vi "BS14P1.vi"() -> ()   [LabVIEW 2019]
doc: "Juego básico de Batalla naval implementado en TCP."
panel:
  out "String":string
  in  "Boolean 54":bool
  in  "Boolean 53":bool
  in  "Boolean 52":bool
  in  "Boolean 51":bool
  in  "?":bool
  out "error out":errorcluster
  in  "Boolean 50":bool
  in  "Boolean 49":bool
  in  "Boolean 48":bool
  in  "Boolean 47":bool
  in  "Boolean 46":bool
  in  "Boolean 45":bool
  in  "Boolean 44":bool
  in  "Boolean 43":bool
  in  "Boolean 42":bool
  in  "Boolean 41":bool
  in  "Boolean 40":bool
  in  "Boolean 39":bool
  in  "Boolean 38":bool
  in  "Boolean 37":bool
  in  "Boolean 36":bool
  in  "Boolean 35":bool
  in  "Boolean 34":bool
  in  "Boolean 33":bool
  in  "Boolean 32":bool
  in  "Boolean 31":bool
  in  "Boolean 30":bool
  in  "Boolean 29":bool
  in  "Boolean 28":bool
  in  "Boolean 27":bool
  in  "Boolean 26":bool
  in  "Boolean 25":bool
  in  "Boolean 24":bool
  in  "Boolean 23":bool
  in  "Boolean 22":bool
  in  "Boolean 21":bool
  in  "Boolean 20":bool
  in  "Boolean 19":bool
  in  "Boolean 18":bool
  in  "Boolean 17":bool
  in  "Boolean 16":bool
  in  "Boolean 15":bool
  in  "Boolean 14":bool
  in  "Boolean 13":bool
  in  "Boolean 12":bool
  in  "Boolean 11":bool
  in  "Boolean 10":bool
  in  "Boolean 9":bool
  in  "Boolean 8":bool
  in  "Boolean 7":bool
  in  "Boolean 6":bool
  in  "Boolean 5":bool
  in  "Boolean 4":bool
  in  "Boolean 3":bool
  in  "Boolean 2":bool
  in  "Boolean":bool
  # "Ship"
  # "Sea"
  # "Hit"
  # "Fail"
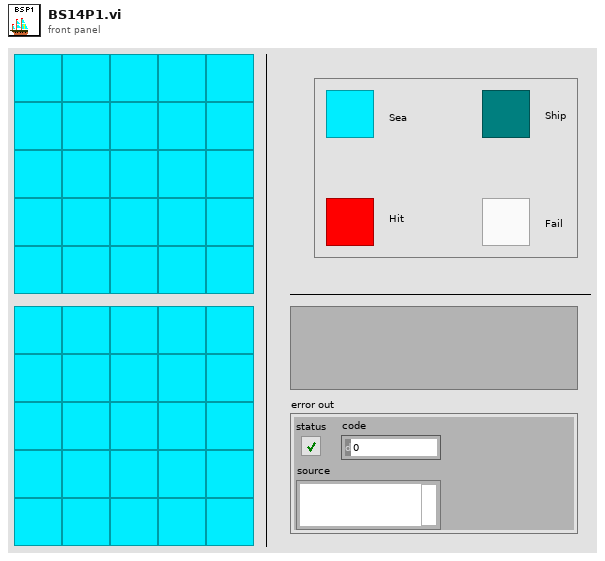
[diagram p1: front panel]
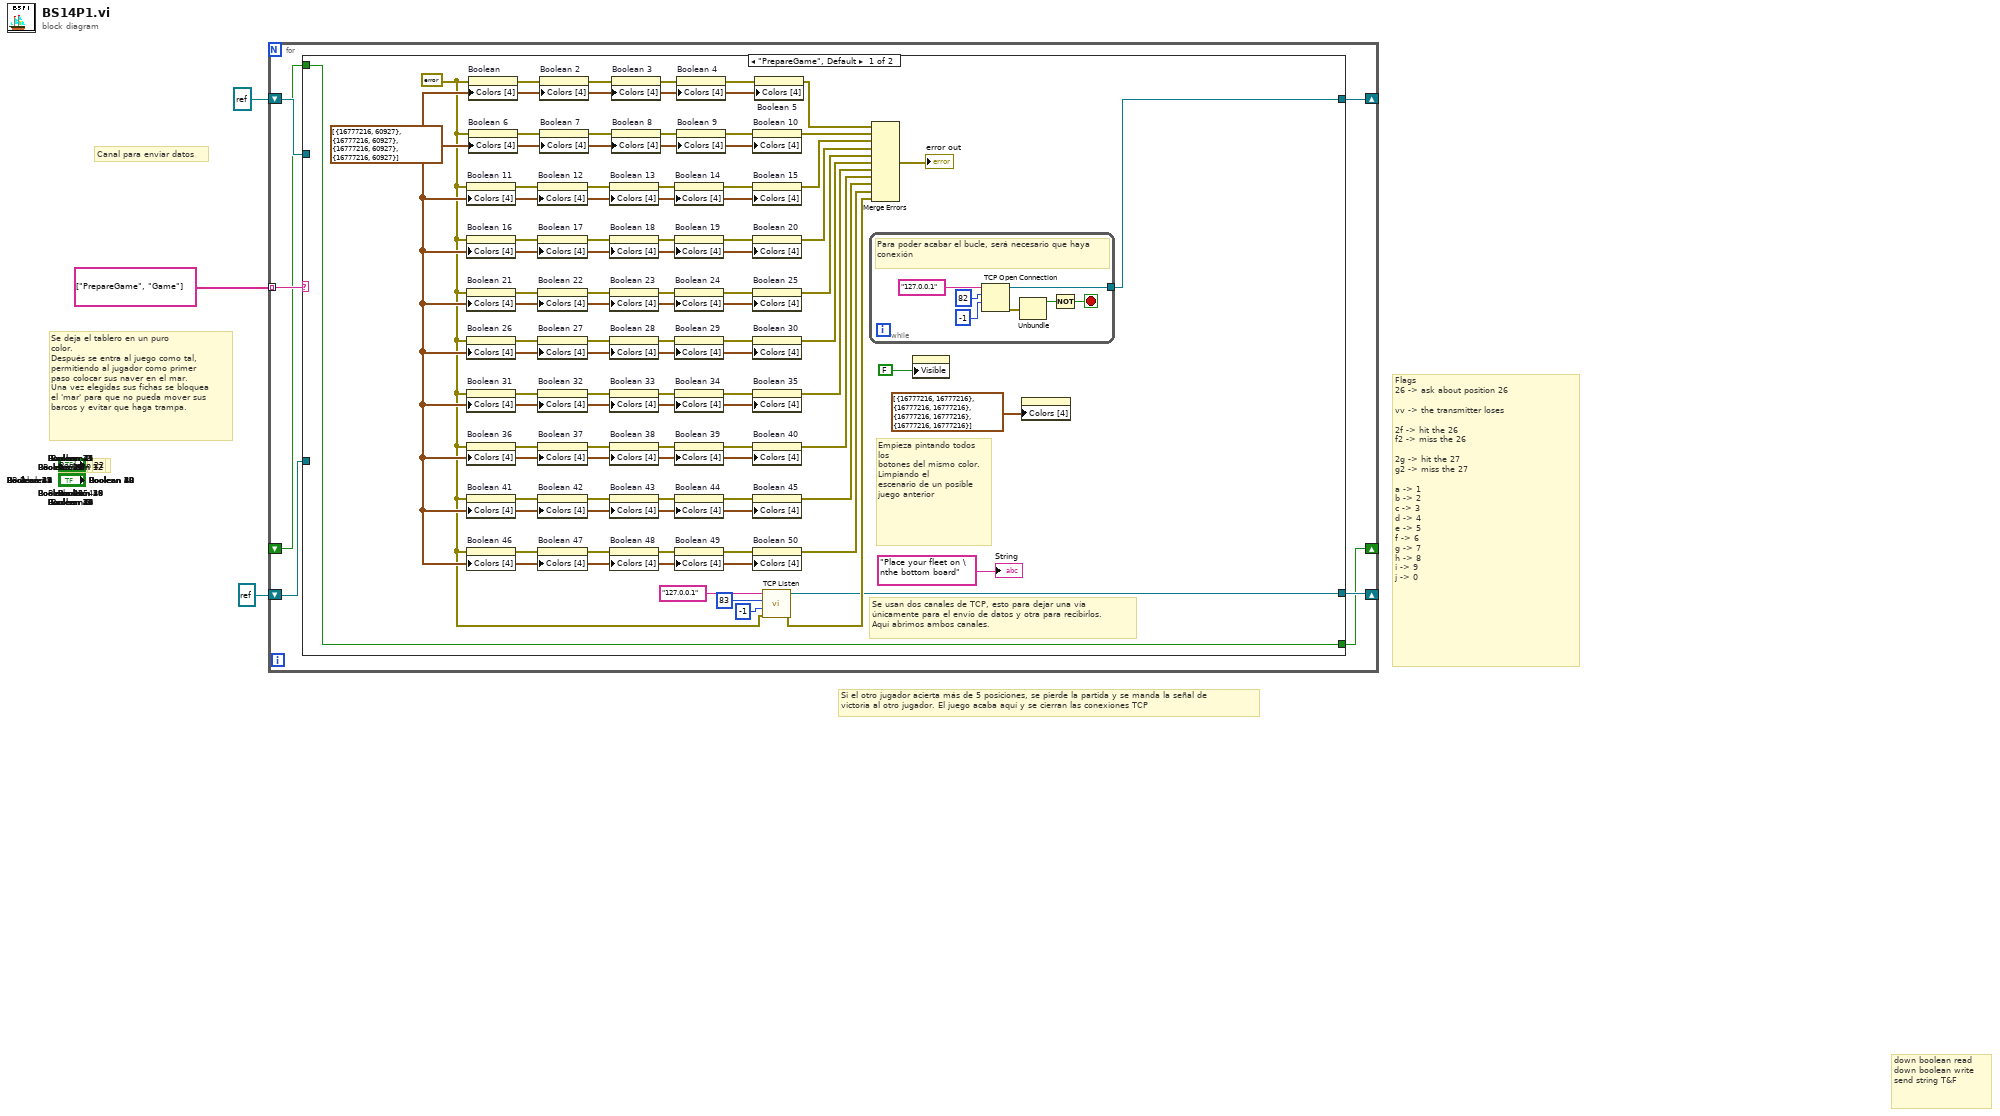
[diagram p0: block diagram]
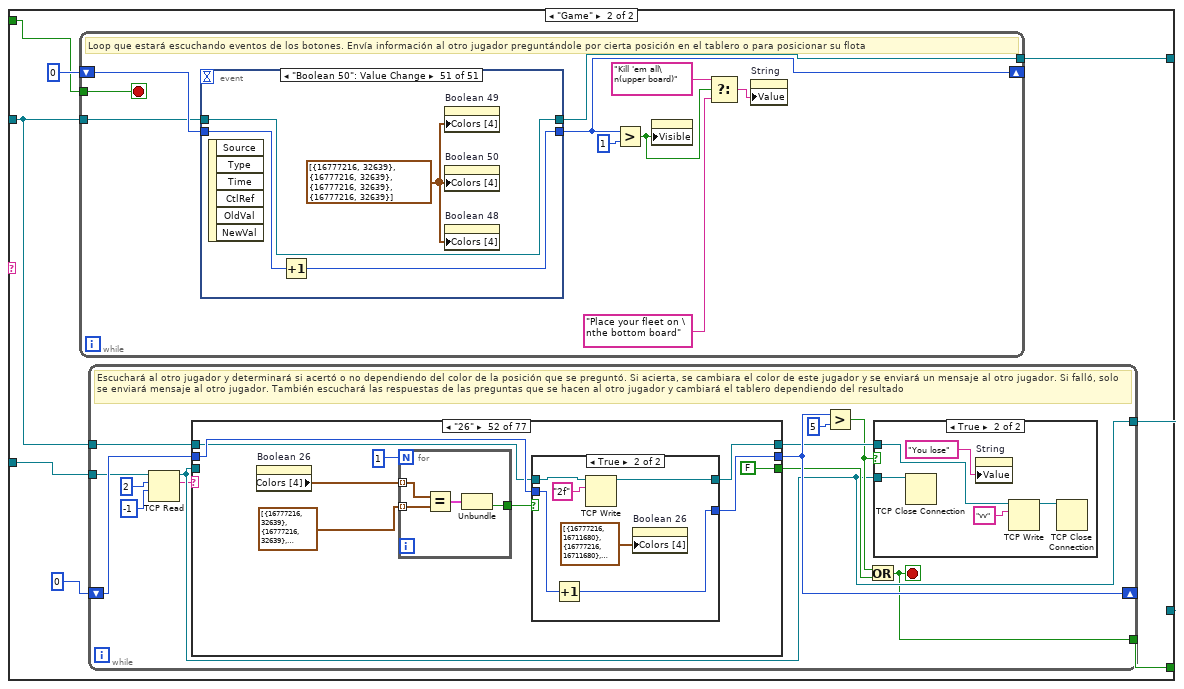
[diagram p2: hidden frame]
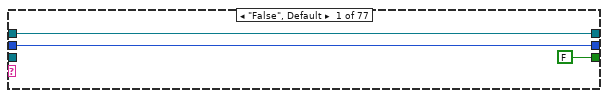
[diagram p3: hidden frame]
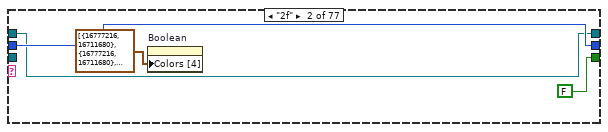
[diagram p4: hidden frame]
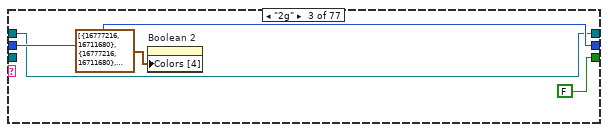
[diagram p5: hidden frame]
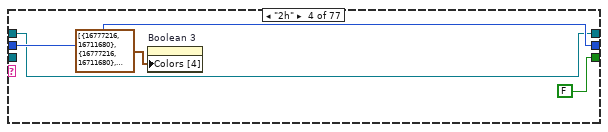
[diagram p6: hidden frame]
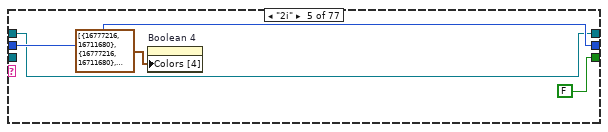
[diagram p7: hidden frame]
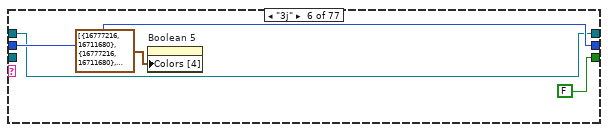
[diagram p8: hidden frame]
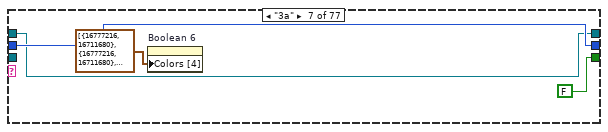
[diagram p9: hidden frame]
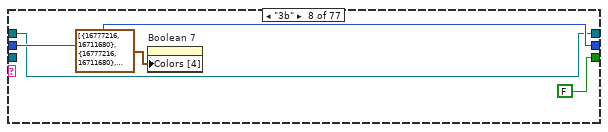
[diagram p10: hidden frame]
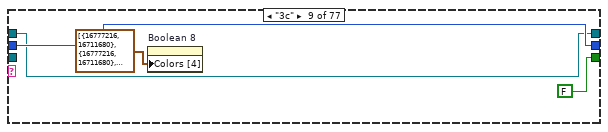
[diagram p11: hidden frame]
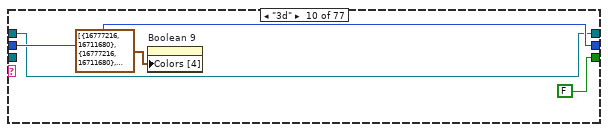
[diagram p12: hidden frame]
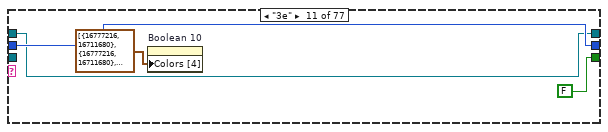
[diagram p13: hidden frame]
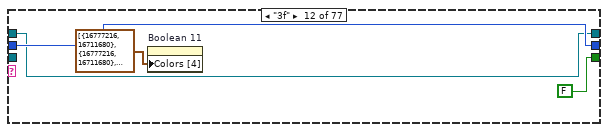
[diagram p14: hidden frame]
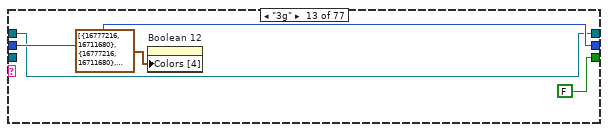
[diagram p15: hidden frame]
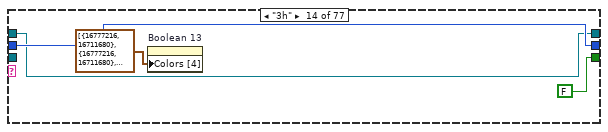
[diagram p16: hidden frame]
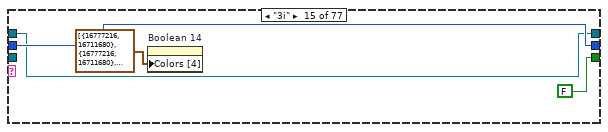
[diagram p17: hidden frame]
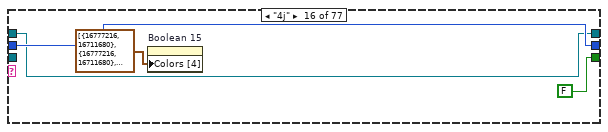
[diagram p18: hidden frame]
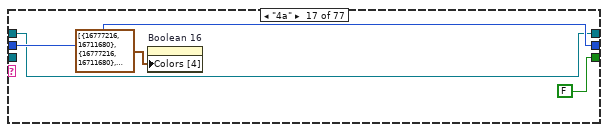
[diagram p19: hidden frame]
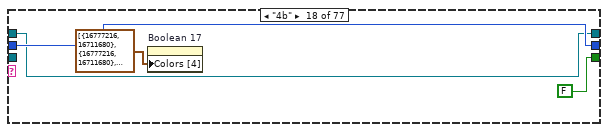
[diagram p20: hidden frame]
diagram:
  # "Si el otro jugador acierta más de 5 posiciones, se pierde la partida y se manda la señal de \nvictoria al otro jugador. El juego acaba aquí y se cierran las conexiones TCP"
  # "Canal para enviar datos"
  # "down boolean read\ndown boolean write \nsend string T&F"
  # "Flags\n26 -> ask about position 26\n\nvv -> the transmitter loses\n\n2f -> hit the 26\nf2 -> miss the 26\n\n2g -> hit the 27\ng2 -> miss the 27 \n\na -> 1\nb -> 2\nc -> 3\nd -> 4\ne -> 5 \nf -> 6 \ng -> 7\nh -> 8\ni -> 9\nj -> 0"
  # "Colors"
  # "block"
  # "Se deja el tablero en un puro \ncolor.\nDespués se entra al juego como tal,\npermitiendo al jugador como primer\npaso colocar sus naver en el mar. \nUna vez elegidas sus fichas se bloquea\nel 'mar' para que no pueda mover sus\nbarcos y evitar que haga trampa."
  # "inferiores"
  # "superiores"
  n1 = for {
    tunnel: string[] ["PrepareGame", "Game"] -> [w10] mode=indexing
    shift-right: [w9] -> _
    shift-left: refnum<k5> refnum ("connection ID") -> [w8]
    shift-right: [w7] -> _
    shift-left: refnum<k5> refnum ("connection ID out") -> [w6]
    shift-right: [w5] -> _
    shift-left: _ -> [w4]
    n2 = case shown="\"PrepareGame\", Default" w10 {
      tunnel: [w13 w84] -> w9
      tunnel: w8 -> [_ w86]
      tunnel: [w12 w85] -> w7
      tunnel: w6 -> [_ w83]
      tunnel: [w11 w82] -> w5
      tunnel: w4 -> [w11 w81]
      frame "PrepareGame", Default {
        w15 = errorcluster {"status"=FALSE, "code"=0, "source"=""} ("error in (no error)")
        w22 = cluster{u32, u32}[] [{16777216, 60927}, {16777216, 60927}, {16777216, 60927}, {16777216, 60927}] ("Colors [4] 2")
        # "Se usan dos canales de TCP, esto para dejar una vía \núnicamente para el envío de datos y otra para recibirlos.\nAquí abrimos ambos canales."
        # "Empieza pintando todos los \nbotones del mismo color. Limpiando el \nescenario de un posible juego anterior"
        n3 = property on="Boolean 11" class="Bool (strict)"(error in=w15, "Colors [4]"=w22) -> (error out=w58:errorcluster)  [unwired: 1 in, 1 out]
        n4 = property on="Boolean 16" class="Bool (strict)"(error in=w15, "Colors [4]"=w22) -> (error out=w56:errorcluster)  [unwired: 1 in, 1 out]
        n5 = property on="Boolean 21" class="Bool (strict)"(error in=w15, "Colors [4]"=w22) -> (error out=w55:errorcluster)  [unwired: 1 in, 1 out]
        n6 = property on="Boolean 26" class="Bool (strict)"(error in=w15, "Colors [4]"=w22) -> (error out=w47:errorcluster)  [unwired: 1 in, 1 out]
        n7 = property on="Boolean 31" class="Bool (strict)"(error in=w15, "Colors [4]"=w22) -> (error out=w43:errorcluster)  [unwired: 1 in, 1 out]
        n8 = property on="Boolean 36" class="Bool (strict)"(error in=w15, "Colors [4]"=w22) -> (error out=w39:errorcluster)  [unwired: 1 in, 1 out]
        n9 = property on="Boolean 41" class="Bool (strict)"(error in=w15, "Colors [4]"=w22) -> (error out=w35:errorcluster)  [unwired: 1 in, 1 out]
        n10 = property on="Boolean 46" class="Bool (strict)"(error in=w15, "Colors [4]"=w22) -> (error out=w31:errorcluster)  [unwired: 1 in, 1 out]
        n11 = property on="Boolean" class="Bool (strict)"(error in=w15, "Colors [4]"=w22) -> (error out=w66:errorcluster)  [unwired: 1 in, 1 out]
        n12 = property on="Boolean 6" class="Bool (strict)"(error in=w15, "Colors [4]"=w22) -> (error out=w62:errorcluster)  [unwired: 1 in, 1 out]
        n13 = property on="Boolean 12" class="Bool (strict)"(error in=w58, "Colors [4]"=w22) -> (error out=w57:errorcluster)  [unwired: 1 in, 1 out]
        n14 = property on="Boolean 17" class="Bool (strict)"(error in=w56, "Colors [4]"=w22) -> (error out=w71:errorcluster)  [unwired: 1 in, 1 out]
        n15 = property on="Boolean 22" class="Bool (strict)"(error in=w55, "Colors [4]"=w22) -> (error out=w68:errorcluster)  [unwired: 1 in, 1 out]
        n16 = property on="Boolean 27" class="Bool (strict)"(error in=w47, "Colors [4]"=w22) -> (error out=w46:errorcluster)  [unwired: 1 in, 1 out]
        n17 = property on="Boolean 32" class="Bool (strict)"(error in=w43, "Colors [4]"=w22) -> (error out=w42:errorcluster)  [unwired: 1 in, 1 out]
        n18 = property on="Boolean 37" class="Bool (strict)"(error in=w39, "Colors [4]"=w22) -> (error out=w38:errorcluster)  [unwired: 1 in, 1 out]
        n19 = property on="Boolean 42" class="Bool (strict)"(error in=w35, "Colors [4]"=w22) -> (error out=w34:errorcluster)  [unwired: 1 in, 1 out]
        n20 = property on="Boolean 47" class="Bool (strict)"(error in=w31, "Colors [4]"=w22) -> (error out=w30:errorcluster)  [unwired: 1 in, 1 out]
        n21 = property on="Boolean 2" class="Bool (strict)"(error in=w66, "Colors [4]"=w22) -> (error out=w65:errorcluster)  [unwired: 1 in, 1 out]
        n22 = property on="Boolean 7" class="Bool (strict)"(error in=w62, "Colors [4]"=w22) -> (error out=w61:errorcluster)  [unwired: 1 in, 1 out]
        n23 = property on="Boolean 13" class="Bool (strict)"(error in=w57, "Colors [4]"=w22) -> (error out=w73:errorcluster)  [unwired: 1 in, 1 out]
        n24 = property on="Boolean 18" class="Bool (strict)"(error in=w71, "Colors [4]"=w22) -> (error out=w70:errorcluster)  [unwired: 1 in, 1 out]
        n25 = property on="Boolean 23" class="Bool (strict)"(error in=w68, "Colors [4]"=w22) -> (error out=w67:errorcluster)  [unwired: 1 in, 1 out]
        n26 = property on="Boolean 28" class="Bool (strict)"(error in=w46, "Colors [4]"=w22) -> (error out=w45:errorcluster)  [unwired: 1 in, 1 out]
        n27 = property on="Boolean 33" class="Bool (strict)"(error in=w42, "Colors [4]"=w22) -> (error out=w41:errorcluster)  [unwired: 1 in, 1 out]
        n28 = property on="Boolean 38" class="Bool (strict)"(error in=w38, "Colors [4]"=w22) -> (error out=w37:errorcluster)  [unwired: 1 in, 1 out]
        n29 = property on="Boolean 43" class="Bool (strict)"(error in=w34, "Colors [4]"=w22) -> (error out=w33:errorcluster)  [unwired: 1 in, 1 out]
        n30 = property on="Boolean 48" class="Bool (strict)"(error in=w30, "Colors [4]"=w22) -> (error out=w29:errorcluster)  [unwired: 1 in, 1 out]
        n31 = property on="Boolean 3" class="Bool (strict)"(error in=w65, "Colors [4]"=w22) -> (error out=w64:errorcluster)  [unwired: 1 in, 1 out]
        n32 = property on="Boolean 8" class="Bool (strict)"(error in=w61, "Colors [4]"=w22) -> (error out=w60:errorcluster)  [unwired: 1 in, 1 out]
        n33 = property on="Boolean 14" class="Bool (strict)"(error in=w73, "Colors [4]"=w22) -> (error out=w72:errorcluster)  [unwired: 1 in, 1 out]
        n34 = property on="Boolean 19" class="Bool (strict)"(error in=w70, "Colors [4]"=w22) -> (error out=w69:errorcluster)  [unwired: 1 in, 1 out]
        n35 = property on="Boolean 24" class="Bool (strict)"(error in=w67, "Colors [4]"=w22) -> (error out=w54:errorcluster)  [unwired: 1 in, 1 out]
        n36 = property on="Boolean 29" class="Bool (strict)"(error in=w45, "Colors [4]"=w22) -> (error out=w44:errorcluster)  [unwired: 1 in, 1 out]
        n37 = property on="Boolean 34" class="Bool (strict)"(error in=w41, "Colors [4]"=w22) -> (error out=w40:errorcluster)  [unwired: 1 in, 1 out]
        n38 = property on="Boolean 39" class="Bool (strict)"(error in=w37, "Colors [4]"=w22) -> (error out=w36:errorcluster)  [unwired: 1 in, 1 out]
        n39 = property on="Boolean 44" class="Bool (strict)"(error in=w33, "Colors [4]"=w22) -> (error out=w32:errorcluster)  [unwired: 1 in, 1 out]
        n40 = property on="Boolean 49" class="Bool (strict)"(error in=w29, "Colors [4]"=w22) -> (error out=w28:errorcluster)  [unwired: 1 in, 1 out]
        n41 = property on="Boolean 4" class="Bool (strict)"(error in=w64, "Colors [4]"=w22) -> (error out=w63:errorcluster)  [unwired: 1 in, 1 out]
        n42 = property on="Boolean 9" class="Bool (strict)"(error in=w60, "Colors [4]"=w22) -> (error out=w59:errorcluster)  [unwired: 1 in, 1 out]
        n43 = property on="Boolean 10" class="Bool (strict)"(error in=w59, "Colors [4]"=w22) -> (error out=w51:errorcluster)  [unwired: 1 in, 1 out]
        n44 = property on="Boolean 15" class="Bool (strict)"(error in=w72, "Colors [4]"=w22) -> (error out=w50:errorcluster)  [unwired: 1 in, 1 out]
        n45 = property on="Boolean 20" class="Bool (strict)"(error in=w69, "Colors [4]"=w22) -> (error out=w49:errorcluster)  [unwired: 1 in, 1 out]
        n46 = property on="Boolean 25" class="Bool (strict)"(error in=w54, "Colors [4]"=w22) -> (error out=w48:errorcluster)  [unwired: 1 in, 1 out]
        n47 = property on="Boolean 30" class="Bool (strict)"(error in=w44, "Colors [4]"=w22) -> (error out=w27:errorcluster)  [unwired: 1 in, 1 out]
        n48 = property on="Boolean 35" class="Bool (strict)"(error in=w40, "Colors [4]"=w22) -> (error out=w26:errorcluster)  [unwired: 1 in, 1 out]
        n49 = property on="Boolean 40" class="Bool (strict)"(error in=w36, "Colors [4]"=w22) -> (error out=w25:errorcluster)  [unwired: 1 in, 1 out]
        n50 = property on="Boolean 45" class="Bool (strict)"(error in=w32, "Colors [4]"=w22) -> (error out=w24:errorcluster)  [unwired: 1 in, 1 out]
        n51 = property on="Boolean 50" class="Bool (strict)"(error in=w28, "Colors [4]"=w22) -> (error out=w23:errorcluster)  [unwired: 1 in, 1 out]
        n52 = property on="Boolean 5" class="Bool (strict)"(error in=w63, "Colors [4]"=w22) -> (error out=w53:errorcluster)  [unwired: 1 in, 1 out]
        n53 = call <vilib>:"TCP Listen.vi"("error in (no error)"=w15, "timeout ms (wait forever: -1)"=-1, "port"=u16 83, "service name"="127.0.0.1") -> ("error out"=w14:errorcluster, "connection ID"=w13:refnum<k5>)  [unwired: 3 in, 3 out]
        n54 = while {
          tunnel: [w74] -> w12
          stop <- w75 stop-if-true
          # "Para poder acabar el bucle, será necesario que haya conexión"
          n55 = TCP Open Connection(address="127.0.0.1", remote port or service name=u16 82, timeout ms (60000)=-1) -> (connection ID=w74:refnum<k5>, error out=w76:errorcluster)  [unwired: 2 in]
          n56 = Unbundle(w76) -> ("status"=w77:bool)  [unwired: 2 out]
          n57 = Not(x=w77) -> (.not. x?=w75:bool)
        }
        n58 = Merge Errors(w53, w51, w50, w49, w48, w27, w26, w25, w24, w23, w14) -> (→"error out":errorcluster)
        n59 = property class="Bool (strict)"("Visible"=FALSE) -> ()  [unwired: 2 in, 2 out]
        n60 = property class="Bool (strict)"("Colors [4]"=cluster{u32, u32}[] [{16777216, 16777216}, {16777216, 16777216}, {16777216, 16777216}, {16777216, 16777216}] ("Colors [4] 2")) -> ()  [unwired: 2 in, 2 out]
        "String" <- "Place your fleet on \nthe bottom board"
      }
      frame "Game" {
        n61 = while {
          shift-right: [w898] -> _
          shift-left: 0 -> [w899]
          tunnel: w83 -> [w892]
          tunnel: [w891] -> w85
          tunnel: w81 -> [w890]
          stop <- w890 stop-if-true
          # "Loop que estará escuchando eventos de los botones. Envía información al otro jugador preguntándole por cierta posición en el tablero o para posicionar su flota"
          n62 = event shown="[50] \"Boolean 50\": Value Change" {
            selector: _ -> [_ _ _ _ _ _ _ _ _ _ _ _ _ _ _ _ _ _ _ _ _ _ _ _ _ _ _ _ _ _ _ _ _ _ _ _ _ _ _ _ _ _ _ _ _ _ _ _ _ _ _]
            dyn-events: _ -> [_ _ _ _ _ _ _ _ _ _ _ _ _ _ _ _ _ _ _ _ _ _ _ _ _ _ _ _ _ _ _ _ _ _ _ _ _ _ _ _ _ _ _ _ _ _ _ _ _ _ _]
            timeout: _ -> [_ _ _ _ _ _ _ _ _ _ _ _ _ _ _ _ _ _ _ _ _ _ _ _ _ _ _ _ _ _ _ _ _ _ _ _ _ _ _ _ _ _ _ _ _ _ _ _ _ _ _]
            tunnel: w899 -> [w901 w905 w909 w913 w917 w921 w925 w929 w933 w937 w941 w945 w949 w953 w957 w961 w965 w969 w973 w977 w981 w985 w989 w993 w997 w1001 w1004 w1008 w1012 w1016 w1020 w1024 w1028 w1032 w1036 w1040 w1044 w1048 w1052 w1056 w1060 w1064 w1068 w1072 w1076 w1080 w1084 w1088 w1092 w1096 w1100]
            tunnel: [w901 w905 w909 w913 w917 w921 w925 w929 w933 w937 w941 w945 w949 w953 w957 w961 w965 w969 w973 w977 w981 w985 w989 w993 w997 w1001 w1003 w1007 w1011 w1015 w1019 w1023 w1027 w1031 w1035 w1039 w1043 w1047 w1051 w1055 w1059 w1063 w1067 w1071 w1075 w1079 w1083 w1087 w1091 w1095 w1099] -> w898
            tunnel: w892 -> [w900 w903 w907 w911 w915 w919 w923 w927 w931 w935 w939 w943 w947 w951 w955 w959 w963 w967 w971 w975 w979 w983 w987 w991 w995 w999 w1002 w1006 w1010 w1014 w1018 w1022 w1026 w1030 w1034 w1038 w1042 w1046 w1050 w1054 w1058 w1062 w1066 w1070 w1074 w1078 w1082 w1086 w1090 w1094 w1098]
            tunnel: [w900 w902 w906 w910 w914 w918 w922 w926 w930 w934 w938 w942 w946 w950 w954 w958 w962 w966 w970 w974 w978 w982 w986 w990 w994 w998 w1002 w1006 w1010 w1014 w1018 w1022 w1026 w1030 w1034 w1038 w1042 w1046 w1050 w1054 w1058 w1062 w1066 w1070 w1074 w1078 w1082 w1086 w1090 w1094 w1098] -> w891
            event Timeout {
              n63 = event-data() -> ()  [unwired: 1 in, 3 out]
            }
            event "Boolean": Value Change {
              n64 = event-data() -> ()  [unwired: 1 in, 6 out]
              n65 = TCP Write(connection ID=w903, data in="26") -> (connection ID out=w902:refnum<k5>)  [unwired: 2 in, 2 out]
            }
            event "Boolean 2": Value Change {
              n66 = event-data() -> ()  [unwired: 1 in, 6 out]
              n67 = TCP Write(connection ID=w907, data in="27") -> (connection ID out=w906:refnum<k5>)  [unwired: 2 in, 2 out]
            }
            event "Boolean 3": Value Change {
              n68 = event-data() -> ()  [unwired: 1 in, 6 out]
              n69 = TCP Write(connection ID=w911, data in="28") -> (connection ID out=w910:refnum<k5>)  [unwired: 2 in, 2 out]
            }
            event "Boolean 4": Value Change {
              n70 = event-data() -> ()  [unwired: 1 in, 6 out]
              n71 = TCP Write(connection ID=w915, data in="29") -> (connection ID out=w914:refnum<k5>)  [unwired: 2 in, 2 out]
            }
            event "Boolean 5": Value Change {
              n72 = event-data() -> ()  [unwired: 1 in, 6 out]
              n73 = TCP Write(connection ID=w919, data in="30") -> (connection ID out=w918:refnum<k5>)  [unwired: 2 in, 2 out]
            }
            event "Boolean 6": Value Change {
              n74 = event-data() -> ()  [unwired: 1 in, 6 out]
              n75 = TCP Write(connection ID=w923, data in="31") -> (connection ID out=w922:refnum<k5>)  [unwired: 2 in, 2 out]
            }
            event "Boolean 7": Value Change {
              n76 = event-data() -> ()  [unwired: 1 in, 6 out]
              n77 = TCP Write(connection ID=w927, data in="32") -> (connection ID out=w926:refnum<k5>)  [unwired: 2 in, 2 out]
            }
            event "Boolean 8": Value Change {
              n78 = event-data() -> ()  [unwired: 1 in, 6 out]
              n79 = TCP Write(connection ID=w931, data in="33") -> (connection ID out=w930:refnum<k5>)  [unwired: 2 in, 2 out]
            }
            event "Boolean 9": Value Change {
              n80 = event-data() -> ()  [unwired: 1 in, 6 out]
              n81 = TCP Write(connection ID=w935, data in="34") -> (connection ID out=w934:refnum<k5>)  [unwired: 2 in, 2 out]
            }
            event "Boolean 10": Value Change {
              n82 = event-data() -> ()  [unwired: 1 in, 6 out]
              n83 = TCP Write(connection ID=w939, data in="35") -> (connection ID out=w938:refnum<k5>)  [unwired: 2 in, 2 out]
            }
            event "Boolean 11": Value Change {
              n84 = event-data() -> ()  [unwired: 1 in, 6 out]
              n85 = TCP Write(connection ID=w943, data in="36") -> (connection ID out=w942:refnum<k5>)  [unwired: 2 in, 2 out]
            }
            event "Boolean 12": Value Change {
              n86 = event-data() -> ()  [unwired: 1 in, 6 out]
              n87 = TCP Write(connection ID=w947, data in="37") -> (connection ID out=w946:refnum<k5>)  [unwired: 2 in, 2 out]
            }
            event "Boolean 13": Value Change {
              n88 = event-data() -> ()  [unwired: 1 in, 6 out]
              n89 = TCP Write(connection ID=w951, data in="38") -> (connection ID out=w950:refnum<k5>)  [unwired: 2 in, 2 out]
            }
            event "Boolean 14": Value Change {
              n90 = event-data() -> ()  [unwired: 1 in, 6 out]
              n91 = TCP Write(connection ID=w955, data in="39") -> (connection ID out=w954:refnum<k5>)  [unwired: 2 in, 2 out]
            }
            event "Boolean 15": Value Change {
              n92 = event-data() -> ()  [unwired: 1 in, 6 out]
              n93 = TCP Write(connection ID=w959, data in="40") -> (connection ID out=w958:refnum<k5>)  [unwired: 2 in, 2 out]
            }
            event "Boolean 16": Value Change {
              n94 = event-data() -> ()  [unwired: 1 in, 6 out]
              n95 = TCP Write(connection ID=w963, data in="41") -> (connection ID out=w962:refnum<k5>)  [unwired: 2 in, 2 out]
            }
            event "Boolean 17": Value Change {
              n96 = event-data() -> ()  [unwired: 1 in, 6 out]
              n97 = TCP Write(connection ID=w967, data in="42") -> (connection ID out=w966:refnum<k5>)  [unwired: 2 in, 2 out]
            }
            event "Boolean 18": Value Change {
              n98 = event-data() -> ()  [unwired: 1 in, 6 out]
              n99 = TCP Write(connection ID=w971, data in="43") -> (connection ID out=w970:refnum<k5>)  [unwired: 2 in, 2 out]
            }
            event "Boolean 19": Value Change {
              n100 = event-data() -> ()  [unwired: 1 in, 6 out]
              n101 = TCP Write(connection ID=w975, data in="44") -> (connection ID out=w974:refnum<k5>)  [unwired: 2 in, 2 out]
            }
            event "Boolean 20": Value Change {
              n102 = event-data() -> ()  [unwired: 1 in, 6 out]
              n103 = TCP Write(connection ID=w979, data in="45") -> (connection ID out=w978:refnum<k5>)  [unwired: 2 in, 2 out]
            }
            event "Boolean 21": Value Change {
              n104 = event-data() -> ()  [unwired: 1 in, 6 out]
              n105 = TCP Write(connection ID=w983, data in="46") -> (connection ID out=w982:refnum<k5>)  [unwired: 2 in, 2 out]
            }
            event "Boolean 22": Value Change {
              n106 = event-data() -> ()  [unwired: 1 in, 6 out]
              n107 = TCP Write(connection ID=w987, data in="47") -> (connection ID out=w986:refnum<k5>)  [unwired: 2 in, 2 out]
            }
            event "Boolean 23": Value Change {
              n108 = event-data() -> ()  [unwired: 1 in, 6 out]
              n109 = TCP Write(connection ID=w991, data in="48") -> (connection ID out=w990:refnum<k5>)  [unwired: 2 in, 2 out]
            }
            event "Boolean 24": Value Change {
              n110 = event-data() -> ()  [unwired: 1 in, 6 out]
              n111 = TCP Write(connection ID=w995, data in="49") -> (connection ID out=w994:refnum<k5>)  [unwired: 2 in, 2 out]
            }
            event "Boolean 25": Value Change {
              n112 = event-data() -> ()  [unwired: 1 in, 6 out]
              n113 = TCP Write(connection ID=w999, data in="50") -> (connection ID out=w998:refnum<k5>)  [unwired: 2 in, 2 out]
            }
            event "Boolean 26": Value Change {
              w1005 = cluster{u32, u32}[] [{16777216, 32639}, {16777216, 32639}, {16777216, 32639}, {16777216, 32639}] ("Colors [4] 2")
              n114 = event-data() -> ()  [unwired: 1 in, 6 out]
              n115 = Increment(x=w1004) -> (x+1=w1003:i32)
              n116 = property on="Boolean 27" class="Bool (strict)"("Colors [4]"=w1005) -> ()  [unwired: 2 in, 2 out]
              n117 = property on="Boolean 28" class="Bool (strict)"("Colors [4]"=w1005) -> ()  [unwired: 2 in, 2 out]
              n118 = property on="Boolean 26" class="Bool (strict)"("Colors [4]"=w1005) -> ()  [unwired: 2 in, 2 out]
            }
            event "Boolean 27": Value Change {
              w1009 = cluster{u32, u32}[] [{16777216, 32639}, {16777216, 32639}, {16777216, 32639}, {16777216, 32639}] ("Colors [4] 2")
              n119 = event-data() -> ()  [unwired: 1 in, 6 out]
              n120 = Increment(x=w1008) -> (x+1=w1007:i32)
              n121 = property on="Boolean 27" class="Bool (strict)"("Colors [4]"=w1009) -> ()  [unwired: 2 in, 2 out]
              n122 = property on="Boolean 28" class="Bool (strict)"("Colors [4]"=w1009) -> ()  [unwired: 2 in, 2 out]
              n123 = property on="Boolean 26" class="Bool (strict)"("Colors [4]"=w1009) -> ()  [unwired: 2 in, 2 out]
            }
            event "Boolean 28": Value Change {
              w1013 = cluster{u32, u32}[] [{16777216, 32639}, {16777216, 32639}, {16777216, 32639}, {16777216, 32639}] ("Colors [4] 2")
              n124 = event-data() -> ()  [unwired: 1 in, 6 out]
              n125 = Increment(x=w1012) -> (x+1=w1011:i32)
              n126 = property on="Boolean 29" class="Bool (strict)"("Colors [4]"=w1013) -> ()  [unwired: 2 in, 2 out]
              n127 = property on="Boolean 27" class="Bool (strict)"("Colors [4]"=w1013) -> ()  [unwired: 2 in, 2 out]
              n128 = property on="Boolean 28" class="Bool (strict)"("Colors [4]"=w1013) -> ()  [unwired: 2 in, 2 out]
            }
            event "Boolean 29": Value Change {
              w1017 = cluster{u32, u32}[] [{16777216, 32639}, {16777216, 32639}, {16777216, 32639}, {16777216, 32639}] ("Colors [4] 2")
              n129 = event-data() -> ()  [unwired: 1 in, 6 out]
              n130 = Increment(x=w1016) -> (x+1=w1015:i32)
              n131 = property on="Boolean 29" class="Bool (strict)"("Colors [4]"=w1017) -> ()  [unwired: 2 in, 2 out]
              n132 = property on="Boolean 30" class="Bool (strict)"("Colors [4]"=w1017) -> ()  [unwired: 2 in, 2 out]
              n133 = property on="Boolean 28" class="Bool (strict)"("Colors [4]"=w1017) -> ()  [unwired: 2 in, 2 out]
            }
            event "Boolean 30": Value Change {
              w1021 = cluster{u32, u32}[] [{16777216, 32639}, {16777216, 32639}, {16777216, 32639}, {16777216, 32639}] ("Colors [4] 2")
              n134 = event-data() -> ()  [unwired: 1 in, 6 out]
              n135 = Increment(x=w1020) -> (x+1=w1019:i32)
              n136 = property on="Boolean 29" class="Bool (strict)"("Colors [4]"=w1021) -> ()  [unwired: 2 in, 2 out]
              n137 = property on="Boolean 30" class="Bool (strict)"("Colors [4]"=w1021) -> ()  [unwired: 2 in, 2 out]
              n138 = property on="Boolean 28" class="Bool (strict)"("Colors [4]"=w1021) -> ()  [unwired: 2 in, 2 out]
            }
            event "Boolean 31": Value Change {
              w1025 = cluster{u32, u32}[] [{16777216, 32639}, {16777216, 32639}, {16777216, 32639}, {16777216, 32639}] ("Colors [4] 2")
              n139 = event-data() -> ()  [unwired: 1 in, 6 out]
              n140 = Increment(x=w1024) -> (x+1=w1023:i32)
              n141 = property on="Boolean 31" class="Bool (strict)"("Colors [4]"=w1025) -> ()  [unwired: 2 in, 2 out]
              n142 = property on="Boolean 32" class="Bool (strict)"("Colors [4]"=w1025) -> ()  [unwired: 2 in, 2 out]
              n143 = property on="Boolean 33" class="Bool (strict)"("Colors [4]"=w1025) -> ()  [unwired: 2 in, 2 out]
            }
            event "Boolean 32": Value Change {
              w1029 = cluster{u32, u32}[] [{16777216, 32639}, {16777216, 32639}, {16777216, 32639}, {16777216, 32639}] ("Colors [4] 2")
              n144 = event-data() -> ()  [unwired: 1 in, 6 out]
              n145 = Increment(x=w1028) -> (x+1=w1027:i32)
              n146 = property on="Boolean 31" class="Bool (strict)"("Colors [4]"=w1029) -> ()  [unwired: 2 in, 2 out]
              n147 = property on="Boolean 32" class="Bool (strict)"("Colors [4]"=w1029) -> ()  [unwired: 2 in, 2 out]
              n148 = property on="Boolean 33" class="Bool (strict)"("Colors [4]"=w1029) -> ()  [unwired: 2 in, 2 out]
            }
            event "Boolean 33": Value Change {
              w1033 = cluster{u32, u32}[] [{16777216, 32639}, {16777216, 32639}, {16777216, 32639}, {16777216, 32639}] ("Colors [4] 2")
              n149 = event-data() -> ()  [unwired: 1 in, 6 out]
              n150 = Increment(x=w1032) -> (x+1=w1031:i32)
              n151 = property on="Boolean 34" class="Bool (strict)"("Colors [4]"=w1033) -> ()  [unwired: 2 in, 2 out]
              n152 = property on="Boolean 32" class="Bool (strict)"("Colors [4]"=w1033) -> ()  [unwired: 2 in, 2 out]
              n153 = property on="Boolean 33" class="Bool (strict)"("Colors [4]"=w1033) -> ()  [unwired: 2 in, 2 out]
            }
            event "Boolean 34": Value Change {
              w1037 = cluster{u32, u32}[] [{16777216, 32639}, {16777216, 32639}, {16777216, 32639}, {16777216, 32639}] ("Colors [4] 2")
              n154 = event-data() -> ()  [unwired: 1 in, 6 out]
              n155 = Increment(x=w1036) -> (x+1=w1035:i32)
              n156 = property on="Boolean 34" class="Bool (strict)"("Colors [4]"=w1037) -> ()  [unwired: 2 in, 2 out]
              n157 = property on="Boolean 35" class="Bool (strict)"("Colors [4]"=w1037) -> ()  [unwired: 2 in, 2 out]
              n158 = property on="Boolean 33" class="Bool (strict)"("Colors [4]"=w1037) -> ()  [unwired: 2 in, 2 out]
            }
            event "Boolean 35": Value Change {
              w1041 = cluster{u32, u32}[] [{16777216, 32639}, {16777216, 32639}, {16777216, 32639}, {16777216, 32639}] ("Colors [4] 2")
              n159 = event-data() -> ()  [unwired: 1 in, 6 out]
              n160 = Increment(x=w1040) -> (x+1=w1039:i32)
              n161 = property on="Boolean 34" class="Bool (strict)"("Colors [4]"=w1041) -> ()  [unwired: 2 in, 2 out]
              n162 = property on="Boolean 35" class="Bool (strict)"("Colors [4]"=w1041) -> ()  [unwired: 2 in, 2 out]
              n163 = property on="Boolean 33" class="Bool (strict)"("Colors [4]"=w1041) -> ()  [unwired: 2 in, 2 out]
            }
            event "Boolean 36": Value Change {
              w1045 = cluster{u32, u32}[] [{16777216, 32639}, {16777216, 32639}, {16777216, 32639}, {16777216, 32639}] ("Colors [4] 2")
              n164 = event-data() -> ()  [unwired: 1 in, 6 out]
              n165 = Increment(x=w1044) -> (x+1=w1043:i32)
              n166 = property on="Boolean 37" class="Bool (strict)"("Colors [4]"=w1045) -> ()  [unwired: 2 in, 2 out]
              n167 = property on="Boolean 38" class="Bool (strict)"("Colors [4]"=w1045) -> ()  [unwired: 2 in, 2 out]
              n168 = property on="Boolean 36" class="Bool (strict)"("Colors [4]"=w1045) -> ()  [unwired: 2 in, 2 out]
            }
            event "Boolean 37": Value Change {
              w1049 = cluster{u32, u32}[] [{16777216, 32639}, {16777216, 32639}, {16777216, 32639}, {16777216, 32639}] ("Colors [4] 2")
              n169 = event-data() -> ()  [unwired: 1 in, 6 out]
              n170 = Increment(x=w1048) -> (x+1=w1047:i32)
              n171 = property on="Boolean 37" class="Bool (strict)"("Colors [4]"=w1049) -> ()  [unwired: 2 in, 2 out]
              n172 = property on="Boolean 38" class="Bool (strict)"("Colors [4]"=w1049) -> ()  [unwired: 2 in, 2 out]
              n173 = property on="Boolean 36" class="Bool (strict)"("Colors [4]"=w1049) -> ()  [unwired: 2 in, 2 out]
            }
            event "Boolean 38": Value Change {
              w1053 = cluster{u32, u32}[] [{16777216, 32639}, {16777216, 32639}, {16777216, 32639}, {16777216, 32639}] ("Colors [4] 2")
              n174 = event-data() -> ()  [unwired: 1 in, 6 out]
              n175 = Increment(x=w1052) -> (x+1=w1051:i32)
              n176 = property on="Boolean 39" class="Bool (strict)"("Colors [4]"=w1053) -> ()  [unwired: 2 in, 2 out]
              n177 = property on="Boolean 38" class="Bool (strict)"("Colors [4]"=w1053) -> ()  [unwired: 2 in, 2 out]
              n178 = property on="Boolean 37" class="Bool (strict)"("Colors [4]"=w1053) -> ()  [unwired: 2 in, 2 out]
            }
            event "Boolean 39": Value Change {
              w1057 = cluster{u32, u32}[] [{16777216, 32639}, {16777216, 32639}, {16777216, 32639}, {16777216, 32639}] ("Colors [4] 2")
              n179 = event-data() -> ()  [unwired: 1 in, 6 out]
              n180 = Increment(x=w1056) -> (x+1=w1055:i32)
              n181 = property on="Boolean 39" class="Bool (strict)"("Colors [4]"=w1057) -> ()  [unwired: 2 in, 2 out]
              n182 = property on="Boolean 40" class="Bool (strict)"("Colors [4]"=w1057) -> ()  [unwired: 2 in, 2 out]
              n183 = property on="Boolean 38" class="Bool (strict)"("Colors [4]"=w1057) -> ()  [unwired: 2 in, 2 out]
            }
            event "Boolean 40": Value Change {
              w1061 = cluster{u32, u32}[] [{16777216, 32639}, {16777216, 32639}, {16777216, 32639}, {16777216, 32639}] ("Colors [4] 2")
              n184 = event-data() -> ()  [unwired: 1 in, 6 out]
              n185 = Increment(x=w1060) -> (x+1=w1059:i32)
              n186 = property on="Boolean 39" class="Bool (strict)"("Colors [4]"=w1061) -> ()  [unwired: 2 in, 2 out]
              n187 = property on="Boolean 40" class="Bool (strict)"("Colors [4]"=w1061) -> ()  [unwired: 2 in, 2 out]
              n188 = property on="Boolean 38" class="Bool (strict)"("Colors [4]"=w1061) -> ()  [unwired: 2 in, 2 out]
            }
            event "Boolean 41": Value Change {
              w1065 = cluster{u32, u32}[] [{16777216, 32639}, {16777216, 32639}, {16777216, 32639}, {16777216, 32639}] ("Colors [4] 2")
              n189 = event-data() -> ()  [unwired: 1 in, 6 out]
              n190 = Increment(x=w1064) -> (x+1=w1063:i32)
              n191 = property on="Boolean 42" class="Bool (strict)"("Colors [4]"=w1065) -> ()  [unwired: 2 in, 2 out]
              n192 = property on="Boolean 43" class="Bool (strict)"("Colors [4]"=w1065) -> ()  [unwired: 2 in, 2 out]
              n193 = property on="Boolean 41" class="Bool (strict)"("Colors [4]"=w1065) -> ()  [unwired: 2 in, 2 out]
            }
            event "Boolean 42": Value Change {
              w1069 = cluster{u32, u32}[] [{16777216, 32639}, {16777216, 32639}, {16777216, 32639}, {16777216, 32639}] ("Colors [4] 2")
              n194 = event-data() -> ()  [unwired: 1 in, 6 out]
              n195 = Increment(x=w1068) -> (x+1=w1067:i32)
              n196 = property on="Boolean 42" class="Bool (strict)"("Colors [4]"=w1069) -> ()  [unwired: 2 in, 2 out]
              n197 = property on="Boolean 43" class="Bool (strict)"("Colors [4]"=w1069) -> ()  [unwired: 2 in, 2 out]
              n198 = property on="Boolean 41" class="Bool (strict)"("Colors [4]"=w1069) -> ()  [unwired: 2 in, 2 out]
            }
            event "Boolean 43": Value Change {
              w1073 = cluster{u32, u32}[] [{16777216, 32639}, {16777216, 32639}, {16777216, 32639}, {16777216, 32639}] ("Colors [4] 2")
              n199 = event-data() -> ()  [unwired: 1 in, 6 out]
              n200 = Increment(x=w1072) -> (x+1=w1071:i32)
              n201 = property on="Boolean 44" class="Bool (strict)"("Colors [4]"=w1073) -> ()  [unwired: 2 in, 2 out]
              n202 = property on="Boolean 43" class="Bool (strict)"("Colors [4]"=w1073) -> ()  [unwired: 2 in, 2 out]
              n203 = property on="Boolean 42" class="Bool (strict)"("Colors [4]"=w1073) -> ()  [unwired: 2 in, 2 out]
            }
            event "Boolean 44": Value Change {
              w1077 = cluster{u32, u32}[] [{16777216, 32639}, {16777216, 32639}, {16777216, 32639}, {16777216, 32639}] ("Colors [4] 2")
              n204 = event-data() -> ()  [unwired: 1 in, 6 out]
              n205 = Increment(x=w1076) -> (x+1=w1075:i32)
              n206 = property on="Boolean 44" class="Bool (strict)"("Colors [4]"=w1077) -> ()  [unwired: 2 in, 2 out]
              n207 = property on="Boolean 45" class="Bool (strict)"("Colors [4]"=w1077) -> ()  [unwired: 2 in, 2 out]
              n208 = property on="Boolean 43" class="Bool (strict)"("Colors [4]"=w1077) -> ()  [unwired: 2 in, 2 out]
            }
            event "Boolean 45": Value Change {
              w1081 = cluster{u32, u32}[] [{16777216, 32639}, {16777216, 32639}, {16777216, 32639}, {16777216, 32639}] ("Colors [4] 2")
              n209 = event-data() -> ()  [unwired: 1 in, 6 out]
              n210 = Increment(x=w1080) -> (x+1=w1079:i32)
              n211 = property on="Boolean 44" class="Bool (strict)"("Colors [4]"=w1081) -> ()  [unwired: 2 in, 2 out]
              n212 = property on="Boolean 45" class="Bool (strict)"("Colors [4]"=w1081) -> ()  [unwired: 2 in, 2 out]
              n213 = property on="Boolean 43" class="Bool (strict)"("Colors [4]"=w1081) -> ()  [unwired: 2 in, 2 out]
            }
            event "Boolean 46": Value Change {
              w1085 = cluster{u32, u32}[] [{16777216, 32639}, {16777216, 32639}, {16777216, 32639}, {16777216, 32639}] ("Colors [4] 2")
              n214 = event-data() -> ()  [unwired: 1 in, 6 out]
              n215 = Increment(x=w1084) -> (x+1=w1083:i32)
              n216 = property on="Boolean 47" class="Bool (strict)"("Colors [4]"=w1085) -> ()  [unwired: 2 in, 2 out]
              n217 = property on="Boolean 48" class="Bool (strict)"("Colors [4]"=w1085) -> ()  [unwired: 2 in, 2 out]
              n218 = property on="Boolean 46" class="Bool (strict)"("Colors [4]"=w1085) -> ()  [unwired: 2 in, 2 out]
            }
            event "Boolean 47": Value Change {
              w1089 = cluster{u32, u32}[] [{16777216, 32639}, {16777216, 32639}, {16777216, 32639}, {16777216, 32639}] ("Colors [4] 2")
              n219 = event-data() -> ()  [unwired: 1 in, 6 out]
              n220 = Increment(x=w1088) -> (x+1=w1087:i32)
              n221 = property on="Boolean 47" class="Bool (strict)"("Colors [4]"=w1089) -> ()  [unwired: 2 in, 2 out]
              n222 = property on="Boolean 48" class="Bool (strict)"("Colors [4]"=w1089) -> ()  [unwired: 2 in, 2 out]
              n223 = property on="Boolean 46" class="Bool (strict)"("Colors [4]"=w1089) -> ()  [unwired: 2 in, 2 out]
            }
            event "Boolean 48": Value Change {
              w1093 = cluster{u32, u32}[] [{16777216, 32639}, {16777216, 32639}, {16777216, 32639}, {16777216, 32639}] ("Colors [4] 2")
              n224 = event-data() -> ()  [unwired: 1 in, 6 out]
              n225 = Increment(x=w1092) -> (x+1=w1091:i32)
              n226 = property on="Boolean 49" class="Bool (strict)"("Colors [4]"=w1093) -> ()  [unwired: 2 in, 2 out]
              n227 = property on="Boolean 48" class="Bool (strict)"("Colors [4]"=w1093) -> ()  [unwired: 2 in, 2 out]
              n228 = property on="Boolean 47" class="Bool (strict)"("Colors [4]"=w1093) -> ()  [unwired: 2 in, 2 out]
            }
            event "Boolean 49": Value Change {
              w1097 = cluster{u32, u32}[] [{16777216, 32639}, {16777216, 32639}, {16777216, 32639}, {16777216, 32639}] ("Colors [4] 2")
              n229 = event-data() -> ()  [unwired: 1 in, 6 out]
              n230 = Increment(x=w1096) -> (x+1=w1095:i32)
              n231 = property on="Boolean 49" class="Bool (strict)"("Colors [4]"=w1097) -> ()  [unwired: 2 in, 2 out]
              n232 = property on="Boolean 50" class="Bool (strict)"("Colors [4]"=w1097) -> ()  [unwired: 2 in, 2 out]
              n233 = property on="Boolean 48" class="Bool (strict)"("Colors [4]"=w1097) -> ()  [unwired: 2 in, 2 out]
            }
            event "Boolean 50": Value Change {
              w1101 = cluster{u32, u32}[] [{16777216, 32639}, {16777216, 32639}, {16777216, 32639}, {16777216, 32639}] ("Colors [4] 2")
              n234 = event-data() -> ()  [unwired: 1 in, 6 out]
              n235 = Increment(x=w1100) -> (x+1=w1099:i32)
              n236 = property on="Boolean 49" class="Bool (strict)"("Colors [4]"=w1101) -> ()  [unwired: 2 in, 2 out]
              n237 = property on="Boolean 50" class="Bool (strict)"("Colors [4]"=w1101) -> ()  [unwired: 2 in, 2 out]
              n238 = property on="Boolean 48" class="Bool (strict)"("Colors [4]"=w1101) -> ()  [unwired: 2 in, 2 out]
            }
          }
          n239 = Greater?(x=w898, y=1) -> (0:w893:bool)
          n240 = property class="Bool (strict)"("Visible"=w893) -> ()  [unwired: 2 in, 2 out]
          n241 = Select(t="Kill 'em all\n(upper board)", s=w893, f="Place your fleet on \nthe bottom board") -> (s? t:f=w894:string)
          n242 = property on="String" class="Str"("Value"=w894) -> ()  [unwired: 2 in, 2 out]
        }
        n243 = while {
          shift-right: [w99] -> _
          shift-left: 0 -> [w100]
          tunnel: w86 -> [w94]
          tunnel: w83 -> [w98]
          tunnel: [w93] -> w84
          tunnel: [w89] -> w82
          stop <- w89 stop-if-true
          # "Escuchará al otro jugador y determinará si acertó o no dependiendo del color de la posición que se preguntó. Si acierta, se cambiara el color de este jugador y se enviará un mensaje al otro jugador. Si falló, solo se enviará mensaje al otro jugador. También escuchará las respuestas de las preguntas que se hacen al otro jugador y cambiará el tablero dependiendo del resultado"
          n244 = TCP Read(connection ID=w94, bytes to read=2, 9:-1 ("timeout ms (25000)")) -> (connection ID out=w93:refnum<k5>, data out=w91:string)  [unwired: 2 in, 1 out]
          n245 = case shown="\"26\"" w91 {
            tunnel: w100 -> [w104 w107 w112 w116 w120 w124 w128 w132 w136 w140 w144 w148 w152 w156 w160 w164 w168 w172 w176 w180 w184 w188 w192 w196 w200 w204 w207 w212 w216 w220 w224 w228 w232 w236 w240 w244 w248 w252 w256 w260 w264 w268 w272 w276 w280 w284 w288 w292 w296 w300 w304 w309 w333 w356 w379 w402 w425 w448 w471 w494 w517 w540 w563 w586 w609 w632 w655 w678 w701 w724 w747 w770 w793 w816 w839 w862 w883]
            tunnel: [w104 w107 w112 w116 w120 w124 w128 w132 w136 w140 w144 w148 w152 w156 w160 w164 w168 w172 w176 w180 w184 w188 w192 w196 w200 w204 w207 w212 w216 w220 w224 w228 w232 w236 w240 w244 w248 w252 w256 w260 w264 w268 w272 w276 w280 w284 w288 w292 w296 w300 w304 w308 w332 w355 w378 w401 w424 w447 w470 w493 w516 w539 w562 w585 w608 w631 w654 w677 w700 w723 w746 w769 w792 w815 w838 w861 w883] -> w99
            tunnel: w93 -> [_ _ _ _ _ _ _ _ _ _ _ _ _ _ _ _ _ _ _ _ _ _ _ _ _ _ _ _ _ _ _ _ _ _ _ _ _ _ _ _ _ _ _ _ _ _ _ _ _ _ _ _ _ _ _ _ _ _ _ _ _ _ _ _ _ _ _ _ _ _ _ _ _ _ _ _ w882]
            tunnel: w98 -> [w103 w106 w110 w114 w118 w122 w126 w130 w134 w138 w142 w146 w150 w154 w158 w162 w166 w170 w174 w178 w182 w186 w190 w194 w198 w202 w206 w210 w214 w218 w222 w226 w230 w234 w238 w242 w246 w250 w254 w258 w262 w266 w270 w274 w278 w282 w286 w290 w294 w298 w302 w307 w330 w353 w376 w399 w422 w445 w468 w491 w514 w537 w560 w583 w606 w629 w652 w675 w698 w721 w744 w767 w790 w813 w836 w859 w881]
            tunnel: [w103 w106 w110 w114 w118 w122 w126 w130 w134 w138 w142 w146 w150 w154 w158 w162 w166 w170 w174 w178 w182 w186 w190 w194 w198 w202 w206 w210 w214 w218 w222 w226 w230 w234 w238 w242 w246 w250 w254 w258 w262 w266 w270 w274 w278 w282 w286 w290 w294 w298 w302 w306 w329 w352 w375 w398 w421 w444 w467 w490 w513 w536 w559 w582 w605 w628 w651 w674 w697 w720 w743 w766 w789 w812 w835 w858 w881] -> w97
            tunnel: [FALSE FALSE FALSE FALSE FALSE FALSE FALSE FALSE FALSE FALSE FALSE FALSE FALSE FALSE FALSE FALSE FALSE FALSE FALSE FALSE FALSE FALSE FALSE FALSE FALSE FALSE FALSE FALSE FALSE FALSE FALSE FALSE FALSE FALSE FALSE FALSE FALSE FALSE FALSE FALSE FALSE FALSE FALSE FALSE FALSE FALSE FALSE FALSE FALSE FALSE FALSE FALSE FALSE FALSE FALSE FALSE FALSE FALSE FALSE FALSE FALSE FALSE FALSE FALSE FALSE FALSE FALSE FALSE FALSE FALSE FALSE FALSE FALSE FALSE FALSE FALSE TRUE] -> w96
            frame "False", Default {
            }
            frame "2f" {
              n246 = property on="Boolean" class="Bool (strict)"("Colors [4]"=cluster{u32, u32}[] [{16777216, 16711680}, {16777216, 16711680}, {16777216, 16711680}, {16777216, 16711680}] ("Colors [4] 2")) -> ()  [unwired: 2 in, 2 out]
            }
            frame "2g" {
              n247 = property on="Boolean 2" class="Bool (strict)"("Colors [4]"=cluster{u32, u32}[] [{16777216, 16711680}, {16777216, 16711680}, {16777216, 16711680}, {16777216, 16711680}] ("Colors [4] 2")) -> ()  [unwired: 2 in, 2 out]
            }
            frame "2h" {
              n248 = property on="Boolean 3" class="Bool (strict)"("Colors [4]"=cluster{u32, u32}[] [{16777216, 16711680}, {16777216, 16711680}, {16777216, 16711680}, {16777216, 16711680}] ("Colors [4] 2")) -> ()  [unwired: 2 in, 2 out]
            }
            frame "2i" {
              n249 = property on="Boolean 4" class="Bool (strict)"("Colors [4]"=cluster{u32, u32}[] [{16777216, 16711680}, {16777216, 16711680}, {16777216, 16711680}, {16777216, 16711680}] ("Colors [4] 2")) -> ()  [unwired: 2 in, 2 out]
            }
            frame "3j" {
              n250 = property on="Boolean 5" class="Bool (strict)"("Colors [4]"=cluster{u32, u32}[] [{16777216, 16711680}, {16777216, 16711680}, {16777216, 16711680}, {16777216, 16711680}] ("Colors [4] 2")) -> ()  [unwired: 2 in, 2 out]
            }
            frame "3a" {
              n251 = property on="Boolean 6" class="Bool (strict)"("Colors [4]"=cluster{u32, u32}[] [{16777216, 16711680}, {16777216, 16711680}, {16777216, 16711680}, {16777216, 16711680}] ("Colors [4] 2")) -> ()  [unwired: 2 in, 2 out]
            }
            frame "3b" {
              n252 = property on="Boolean 7" class="Bool (strict)"("Colors [4]"=cluster{u32, u32}[] [{16777216, 16711680}, {16777216, 16711680}, {16777216, 16711680}, {16777216, 16711680}] ("Colors [4] 2")) -> ()  [unwired: 2 in, 2 out]
            }
            frame "3c" {
              n253 = property on="Boolean 8" class="Bool (strict)"("Colors [4]"=cluster{u32, u32}[] [{16777216, 16711680}, {16777216, 16711680}, {16777216, 16711680}, {16777216, 16711680}] ("Colors [4] 2")) -> ()  [unwired: 2 in, 2 out]
            }
            frame "3d" {
              n254 = property on="Boolean 9" class="Bool (strict)"("Colors [4]"=cluster{u32, u32}[] [{16777216, 16711680}, {16777216, 16711680}, {16777216, 16711680}, {16777216, 16711680}] ("Colors [4] 2")) -> ()  [unwired: 2 in, 2 out]
            }
            frame "3e" {
              n255 = property on="Boolean 10" class="Bool (strict)"("Colors [4]"=cluster{u32, u32}[] [{16777216, 16711680}, {16777216, 16711680}, {16777216, 16711680}, {16777216, 16711680}] ("Colors [4] 2")) -> ()  [unwired: 2 in, 2 out]
            }
            frame "3f" {
              n256 = property on="Boolean 11" class="Bool (strict)"("Colors [4]"=cluster{u32, u32}[] [{16777216, 16711680}, {16777216, 16711680}, {16777216, 16711680}, {16777216, 16711680}] ("Colors [4] 2")) -> ()  [unwired: 2 in, 2 out]
            }
            frame "3g" {
              n257 = property on="Boolean 12" class="Bool (strict)"("Colors [4]"=cluster{u32, u32}[] [{16777216, 16711680}, {16777216, 16711680}, {16777216, 16711680}, {16777216, 16711680}] ("Colors [4] 2")) -> ()  [unwired: 2 in, 2 out]
            }
            frame "3h" {
              n258 = property on="Boolean 13" class="Bool (strict)"("Colors [4]"=cluster{u32, u32}[] [{16777216, 16711680}, {16777216, 16711680}, {16777216, 16711680}, {16777216, 16711680}] ("Colors [4] 2")) -> ()  [unwired: 2 in, 2 out]
            }
            frame "3i" {
              n259 = property on="Boolean 14" class="Bool (strict)"("Colors [4]"=cluster{u32, u32}[] [{16777216, 16711680}, {16777216, 16711680}, {16777216, 16711680}, {16777216, 16711680}] ("Colors [4] 2")) -> ()  [unwired: 2 in, 2 out]
            }
            frame "4j" {
              n260 = property on="Boolean 15" class="Bool (strict)"("Colors [4]"=cluster{u32, u32}[] [{16777216, 16711680}, {16777216, 16711680}, {16777216, 16711680}, {16777216, 16711680}] ("Colors [4] 2")) -> ()  [unwired: 2 in, 2 out]
            }
            frame "4a" {
              n261 = property on="Boolean 16" class="Bool (strict)"("Colors [4]"=cluster{u32, u32}[] [{16777216, 16711680}, {16777216, 16711680}, {16777216, 16711680}, {16777216, 16711680}] ("Colors [4] 2")) -> ()  [unwired: 2 in, 2 out]
            }
            frame "4b" {
              n262 = property on="Boolean 17" class="Bool (strict)"("Colors [4]"=cluster{u32, u32}[] [{16777216, 16711680}, {16777216, 16711680}, {16777216, 16711680}, {16777216, 16711680}] ("Colors [4] 2")) -> ()  [unwired: 2 in, 2 out]
            }
            frame "4c" {
              n263 = property on="Boolean 18" class="Bool (strict)"("Colors [4]"=cluster{u32, u32}[] [{16777216, 16711680}, {16777216, 16711680}, {16777216, 16711680}, {16777216, 16711680}] ("Colors [4] 2")) -> ()  [unwired: 2 in, 2 out]
            }
            frame "4d" {
              n264 = property on="Boolean 19" class="Bool (strict)"("Colors [4]"=cluster{u32, u32}[] [{16777216, 16711680}, {16777216, 16711680}, {16777216, 16711680}, {16777216, 16711680}] ("Colors [4] 2")) -> ()  [unwired: 2 in, 2 out]
            }
            frame "4e" {
              n265 = property on="Boolean 20" class="Bool (strict)"("Colors [4]"=cluster{u32, u32}[] [{16777216, 16711680}, {16777216, 16711680}, {16777216, 16711680}, {16777216, 16711680}] ("Colors [4] 2")) -> ()  [unwired: 2 in, 2 out]
            }
            frame "4f" {
              n266 = property on="Boolean 21" class="Bool (strict)"("Colors [4]"=cluster{u32, u32}[] [{16777216, 16711680}, {16777216, 16711680}, {16777216, 16711680}, {16777216, 16711680}] ("Colors [4] 2")) -> ()  [unwired: 2 in, 2 out]
            }
            frame "4g" {
              n267 = property on="Boolean 22" class="Bool (strict)"("Colors [4]"=cluster{u32, u32}[] [{16777216, 16711680}, {16777216, 16711680}, {16777216, 16711680}, {16777216, 16711680}] ("Colors [4] 2")) -> ()  [unwired: 2 in, 2 out]
            }
            frame "4h" {
              n268 = property on="Boolean 23" class="Bool (strict)"("Colors [4]"=cluster{u32, u32}[] [{16777216, 16711680}, {16777216, 16711680}, {16777216, 16711680}, {16777216, 16711680}] ("Colors [4] 2")) -> ()  [unwired: 2 in, 2 out]
            }
            frame "4i" {
              n269 = property on="Boolean 24" class="Bool (strict)"("Colors [4]"=cluster{u32, u32}[] [{16777216, 16711680}, {16777216, 16711680}, {16777216, 16711680}, {16777216, 16711680}] ("Colors [4] 2")) -> ()  [unwired: 2 in, 2 out]
            }
            frame "5j" {
              n270 = property on="Boolean 25" class="Bool (strict)"("Colors [4]"=cluster{u32, u32}[] [{16777216, 16711680}, {16777216, 16711680}, {16777216, 16711680}, {16777216, 16711680}] ("Colors [4] 2")) -> ()  [unwired: 2 in, 2 out]
            }
            frame "f2" {
              n271 = property on="Boolean" class="Bool (strict)"("Colors [4]"=cluster{u32, u32}[] [{16777216, 16448250}, {16777216, 16448250}, {16777216, 16448250}, {16777216, 16448250}] ("Colors [4] 2")) -> ()  [unwired: 2 in, 2 out]
            }
            frame "g2" {
              n272 = property on="Boolean 2" class="Bool (strict)"("Colors [4]"=cluster{u32, u32}[] [{16777216, 16448250}, {16777216, 16448250}, {16777216, 16448250}, {16777216, 16448250}] ("Colors [4] 2")) -> ()  [unwired: 2 in, 2 out]
            }
            frame "h2" {
              n273 = property on="Boolean 3" class="Bool (strict)"("Colors [4]"=cluster{u32, u32}[] [{16777216, 16448250}, {16777216, 16448250}, {16777216, 16448250}, {16777216, 16448250}] ("Colors [4] 2")) -> ()  [unwired: 2 in, 2 out]
            }
            frame "i2" {
              n274 = property on="Boolean 4" class="Bool (strict)"("Colors [4]"=cluster{u32, u32}[] [{16777216, 16448250}, {16777216, 16448250}, {16777216, 16448250}, {16777216, 16448250}] ("Colors [4] 2")) -> ()  [unwired: 2 in, 2 out]
            }
            frame "j3" {
              n275 = property on="Boolean 5" class="Bool (strict)"("Colors [4]"=cluster{u32, u32}[] [{16777216, 16448250}, {16777216, 16448250}, {16777216, 16448250}, {16777216, 16448250}] ("Colors [4] 2")) -> ()  [unwired: 2 in, 2 out]
            }
            frame "a3" {
              n276 = property on="Boolean 6" class="Bool (strict)"("Colors [4]"=cluster{u32, u32}[] [{16777216, 16448250}, {16777216, 16448250}, {16777216, 16448250}, {16777216, 16448250}] ("Colors [4] 2")) -> ()  [unwired: 2 in, 2 out]
            }
            frame "b3" {
              n277 = property on="Boolean 7" class="Bool (strict)"("Colors [4]"=cluster{u32, u32}[] [{16777216, 16448250}, {16777216, 16448250}, {16777216, 16448250}, {16777216, 16448250}] ("Colors [4] 2")) -> ()  [unwired: 2 in, 2 out]
            }
            frame "c3" {
              n278 = property on="Boolean 8" class="Bool (strict)"("Colors [4]"=cluster{u32, u32}[] [{16777216, 16448250}, {16777216, 16448250}, {16777216, 16448250}, {16777216, 16448250}] ("Colors [4] 2")) -> ()  [unwired: 2 in, 2 out]
            }
            frame "d3" {
              n279 = property on="Boolean 9" class="Bool (strict)"("Colors [4]"=cluster{u32, u32}[] [{16777216, 16448250}, {16777216, 16448250}, {16777216, 16448250}, {16777216, 16448250}] ("Colors [4] 2")) -> ()  [unwired: 2 in, 2 out]
            }
            frame "e3" {
              n280 = property on="Boolean 10" class="Bool (strict)"("Colors [4]"=cluster{u32, u32}[] [{16777216, 16448250}, {16777216, 16448250}, {16777216, 16448250}, {16777216, 16448250}] ("Colors [4] 2")) -> ()  [unwired: 2 in, 2 out]
            }
            frame "f3" {
              n281 = property on="Boolean 11" class="Bool (strict)"("Colors [4]"=cluster{u32, u32}[] [{16777216, 16448250}, {16777216, 16448250}, {16777216, 16448250}, {16777216, 16448250}] ("Colors [4] 2")) -> ()  [unwired: 2 in, 2 out]
            }
            frame "g3" {
              n282 = property on="Boolean 12" class="Bool (strict)"("Colors [4]"=cluster{u32, u32}[] [{16777216, 16448250}, {16777216, 16448250}, {16777216, 16448250}, {16777216, 16448250}] ("Colors [4] 2")) -> ()  [unwired: 2 in, 2 out]
            }
            frame "h3" {
              n283 = property on="Boolean 13" class="Bool (strict)"("Colors [4]"=cluster{u32, u32}[] [{16777216, 16448250}, {16777216, 16448250}, {16777216, 16448250}, {16777216, 16448250}] ("Colors [4] 2")) -> ()  [unwired: 2 in, 2 out]
            }
            frame "i3" {
              n284 = property on="Boolean 14" class="Bool (strict)"("Colors [4]"=cluster{u32, u32}[] [{16777216, 16448250}, {16777216, 16448250}, {16777216, 16448250}, {16777216, 16448250}] ("Colors [4] 2")) -> ()  [unwired: 2 in, 2 out]
            }
            frame "j4" {
              n285 = property on="Boolean 15" class="Bool (strict)"("Colors [4]"=cluster{u32, u32}[] [{16777216, 16448250}, {16777216, 16448250}, {16777216, 16448250}, {16777216, 16448250}] ("Colors [4] 2")) -> ()  [unwired: 2 in, 2 out]
            }
            frame "a4" {
              n286 = property on="Boolean 16" class="Bool (strict)"("Colors [4]"=cluster{u32, u32}[] [{16777216, 16448250}, {16777216, 16448250}, {16777216, 16448250}, {16777216, 16448250}] ("Colors [4] 2")) -> ()  [unwired: 2 in, 2 out]
            }
            frame "b4" {
              n287 = property on="Boolean 17" class="Bool (strict)"("Colors [4]"=cluster{u32, u32}[] [{16777216, 16448250}, {16777216, 16448250}, {16777216, 16448250}, {16777216, 16448250}] ("Colors [4] 2")) -> ()  [unwired: 2 in, 2 out]
            }
            frame "c4" {
              n288 = property on="Boolean 18" class="Bool (strict)"("Colors [4]"=cluster{u32, u32}[] [{16777216, 16448250}, {16777216, 16448250}, {16777216, 16448250}, {16777216, 16448250}] ("Colors [4] 2")) -> ()  [unwired: 2 in, 2 out]
            }
            frame "d4" {
              n289 = property on="Boolean 19" class="Bool (strict)"("Colors [4]"=cluster{u32, u32}[] [{16777216, 16448250}, {16777216, 16448250}, {16777216, 16448250}, {16777216, 16448250}] ("Colors [4] 2")) -> ()  [unwired: 2 in, 2 out]
            }
            frame "e4" {
              n290 = property on="Boolean 20" class="Bool (strict)"("Colors [4]"=cluster{u32, u32}[] [{16777216, 16448250}, {16777216, 16448250}, {16777216, 16448250}, {16777216, 16448250}] ("Colors [4] 2")) -> ()  [unwired: 2 in, 2 out]
            }
            frame "f4" {
              n291 = property on="Boolean 21" class="Bool (strict)"("Colors [4]"=cluster{u32, u32}[] [{16777216, 16448250}, {16777216, 16448250}, {16777216, 16448250}, {16777216, 16448250}] ("Colors [4] 2")) -> ()  [unwired: 2 in, 2 out]
            }
            frame "g4" {
              n292 = property on="Boolean 22" class="Bool (strict)"("Colors [4]"=cluster{u32, u32}[] [{16777216, 16448250}, {16777216, 16448250}, {16777216, 16448250}, {16777216, 16448250}] ("Colors [4] 2")) -> ()  [unwired: 2 in, 2 out]
            }
            frame "h4" {
              n293 = property on="Boolean 23" class="Bool (strict)"("Colors [4]"=cluster{u32, u32}[] [{16777216, 16448250}, {16777216, 16448250}, {16777216, 16448250}, {16777216, 16448250}] ("Colors [4] 2")) -> ()  [unwired: 2 in, 2 out]
            }
            frame "i4" {
              n294 = property on="Boolean 24" class="Bool (strict)"("Colors [4]"=cluster{u32, u32}[] [{16777216, 16448250}, {16777216, 16448250}, {16777216, 16448250}, {16777216, 16448250}] ("Colors [4] 2")) -> ()  [unwired: 2 in, 2 out]
            }
            frame "j5" {
              n295 = property on="Boolean 25" class="Bool (strict)"("Colors [4]"=cluster{u32, u32}[] [{16777216, 16448250}, {16777216, 16448250}, {16777216, 16448250}, {16777216, 16448250}] ("Colors [4] 2")) -> ()  [unwired: 2 in, 2 out]
            }
            frame "26" {
              n296 = property on="Boolean 26" class="Bool (strict)"() -> ("Colors [4]"=w312:cluster{u32, u32}[])  [unwired: 2 in, 2 out]
              n297 = for {
                N: 1 -> [_]
                tunnel: w312 -> [w327] mode=indexing
                tunnel: cluster{u32, u32}[] [{16777216, 32639}, {16777216, 32639}, {16777216, 32639}, {16777216, 32639}] ("Colors [4] 2") -> [w326] mode=indexing
                tunnel: [w324] -> w310
                n298 = Equal?(x=w327, y=w326) -> (x = y?=w325:cluster{bool, bool})
                n299 = Unbundle(w325) -> (w324:bool)  [unwired: 1 out]
              }
              n300 = case shown="True" w310 {
                tunnel: w309 -> [w317 w322]
                tunnel: [w317 w321] -> w308
                tunnel: w307 -> [w315 w320]
                tunnel: [w314 w318] -> w306
                frame False {
                  n301 = TCP Write(connection ID=w315, data in="f2") -> (connection ID out=w314:refnum<k5>)  [unwired: 2 in, 2 out]
                }
                frame True {
                  n302 = Increment(x=w322) -> (x+1=w321:i32)
                  n303 = TCP Write(connection ID=w320, data in="2f") -> (connection ID out=w318:refnum<k5>)  [unwired: 2 in, 2 out]
                  n304 = property on="Boolean 26" class="Bool (strict)"("Colors [4]"=cluster{u32, u32}[] [{16777216, 16711680}, {16777216, 16711680}, {16777216, 16711680}, {16777216, 16711680}] ("Colors [4] 2")) -> ()  [unwired: 2 in, 2 out]
                }
              }
            }
            frame "27" {
              n305 = property on="Boolean 27" class="Bool (strict)"() -> ("Colors [4]"=w331:cluster{u32, u32}[])  [unwired: 2 in, 2 out]
              n306 = for {
                N: 1 -> [_]
                tunnel: w331 -> [w350] mode=indexing
                tunnel: cluster{u32, u32}[] [{16777216, 32639}, {16777216, 32639}, {16777216, 32639}, {16777216, 32639}] ("Colors [4] 2") -> [w349] mode=indexing
                tunnel: [w347] -> w334
                n307 = Equal?(x=w350, y=w349) -> (x = y?=w348:cluster{bool, bool})
                n308 = Unbundle(w348) -> (w347:bool)  [unwired: 1 out]
              }
              n309 = case shown="False" w334 {
                tunnel: w333 -> [w340 w346]
                tunnel: [w340 w345] -> w332
                tunnel: w330 -> [w338 w342]
                tunnel: [w337 w341] -> w329
                frame False {
                  (unwired) u16 82 ("port")
                  n310 = TCP Write(connection ID=w338, data in="g2") -> (connection ID out=w337:refnum<k5>)  [unwired: 2 in, 2 out]
                }
                frame True {
                  n311 = TCP Write(connection ID=w342, data in="2g") -> (connection ID out=w341:refnum<k5>)  [unwired: 2 in, 2 out]
                  n312 = Increment(x=w346) -> (x+1=w345:i32)
                  n313 = property on="Boolean 27" class="Bool (strict)"("Colors [4]"=cluster{u32, u32}[] [{16777216, 16711680}, {16777216, 16711680}, {16777216, 16711680}, {16777216, 16711680}] ("Colors [4] 2")) -> ()  [unwired: 2 in, 2 out]
                }
              }
            }
            frame "28" {
              n314 = property on="Boolean 28" class="Bool (strict)"() -> ("Colors [4]"=w354:cluster{u32, u32}[])  [unwired: 2 in, 2 out]
              n315 = for {
                N: 1 -> [_]
                tunnel: w354 -> [w373] mode=indexing
                tunnel: cluster{u32, u32}[] [{16777216, 32639}, {16777216, 32639}, {16777216, 32639}, {16777216, 32639}] ("Colors [4] 2") -> [w372] mode=indexing
                tunnel: [w370] -> w357
                n316 = Equal?(x=w373, y=w372) -> (x = y?=w371:cluster{bool, bool})
                n317 = Unbundle(w371) -> (w370:bool)  [unwired: 1 out]
              }
              n318 = case shown="False" w357 {
                tunnel: w356 -> [w363 w369]
                tunnel: [w363 w368] -> w355
                tunnel: w353 -> [w361 w365]
                tunnel: [w360 w366] -> w352
                frame False {
                  n319 = TCP Write(connection ID=w361, data in="h2") -> (connection ID out=w360:refnum<k5>)  [unwired: 2 in, 2 out]
                }
                frame True {
                  n320 = Increment(x=w369) -> (x+1=w368:i32)
                  n321 = TCP Write(connection ID=w365, data in="2h") -> (connection ID out=w366:refnum<k5>)  [unwired: 2 in, 2 out]
                  n322 = property on="Boolean 28" class="Bool (strict)"("Colors [4]"=cluster{u32, u32}[] [{16777216, 16711680}, {16777216, 16711680}, {16777216, 16711680}, {16777216, 16711680}] ("Colors [4] 2")) -> ()  [unwired: 2 in, 2 out]
                }
              }
            }
            frame "29" {
              n323 = property on="Boolean 29" class="Bool (strict)"() -> ("Colors [4]"=w377:cluster{u32, u32}[])  [unwired: 2 in, 2 out]
              n324 = for {
                N: 1 -> [_]
                tunnel: cluster{u32, u32}[] [{16777216, 32639}, {16777216, 32639}, {16777216, 32639}, {16777216, 32639}] ("Colors [4] 2") -> [w396] mode=indexing
                tunnel: [w394] -> w380
                tunnel: w377 -> [w393] mode=indexing
                n325 = Equal?(x=w393, y=w396) -> (x = y?=w395:cluster{bool, bool})
                n326 = Unbundle(w395) -> (w394:bool)  [unwired: 1 out]
              }
              n327 = case shown="True" w380 {
                tunnel: w379 -> [w386 w392]
                tunnel: [w386 w391] -> w378
                tunnel: w376 -> [w384 w389]
                tunnel: [w383 w387] -> w375
                frame False {
                  n328 = TCP Write(connection ID=w384, data in="i2") -> (connection ID out=w383:refnum<k5>)  [unwired: 2 in, 2 out]
                }
                frame True {
                  n329 = Increment(x=w392) -> (x+1=w391:i32)
                  n330 = TCP Write(connection ID=w389, data in="2i") -> (connection ID out=w387:refnum<k5>)  [unwired: 2 in, 2 out]
                  n331 = property on="Boolean 29" class="Bool (strict)"("Colors [4]"=cluster{u32, u32}[] [{16777216, 16711680}, {16777216, 16711680}, {16777216, 16711680}, {16777216, 16711680}] ("Colors [4] 2")) -> ()  [unwired: 2 in, 2 out]
                }
              }
            }
            frame "30" {
              n332 = property on="Boolean 30" class="Bool (strict)"() -> ("Colors [4]"=w400:cluster{u32, u32}[])  [unwired: 2 in, 2 out]
              n333 = for {
                N: 1 -> [_]
                tunnel: cluster{u32, u32}[] [{16777216, 32639}, {16777216, 32639}, {16777216, 32639}, {16777216, 32639}] ("Colors [4] 2") -> [w419] mode=indexing
                tunnel: [w417] -> w403
                tunnel: w400 -> [w416] mode=indexing
                n334 = Equal?(x=w416, y=w419) -> (x = y?=w418:cluster{bool, bool})
                n335 = Unbundle(w418) -> (w417:bool)  [unwired: 1 out]
              }
              n336 = case shown="True" w403 {
                tunnel: w402 -> [w409 w415]
                tunnel: [w409 w414] -> w401
                tunnel: w399 -> [w407 w411]
                tunnel: [w406 w410] -> w398
                frame False {
                  n337 = TCP Write(connection ID=w407, data in="j3") -> (connection ID out=w406:refnum<k5>)  [unwired: 2 in, 2 out]
                }
                frame True {
                  n338 = Increment(x=w415) -> (x+1=w414:i32)
                  n339 = TCP Write(connection ID=w411, data in="3j") -> (connection ID out=w410:refnum<k5>)  [unwired: 2 in, 2 out]
                  n340 = property on="Boolean 30" class="Bool (strict)"("Colors [4]"=cluster{u32, u32}[] [{16777216, 16711680}, {16777216, 16711680}, {16777216, 16711680}, {16777216, 16711680}] ("Colors [4] 2")) -> ()  [unwired: 2 in, 2 out]
                }
              }
            }
            frame "31" {
              n341 = property on="Boolean 31" class="Bool (strict)"() -> ("Colors [4]"=w423:cluster{u32, u32}[])  [unwired: 2 in, 2 out]
              n342 = for {
                N: 1 -> [_]
                tunnel: cluster{u32, u32}[] [{16777216, 32639}, {16777216, 32639}, {16777216, 32639}, {16777216, 32639}] ("Colors [4] 2") -> [w442] mode=indexing
                tunnel: [w440] -> w426
                tunnel: w423 -> [w439] mode=indexing
                n343 = Equal?(x=w439, y=w442) -> (x = y?=w441:cluster{bool, bool})
                n344 = Unbundle(w441) -> (w440:bool)  [unwired: 1 out]
              }
              n345 = case shown="True" w426 {
                tunnel: w425 -> [w432 w438]
                tunnel: [w432 w437] -> w424
                tunnel: w422 -> [w430 w435]
                tunnel: [w429 w433] -> w421
                frame False {
                  n346 = TCP Write(connection ID=w430, data in="a3") -> (connection ID out=w429:refnum<k5>)  [unwired: 2 in, 2 out]
                }
                frame True {
                  n347 = Increment(x=w438) -> (x+1=w437:i32)
                  n348 = TCP Write(connection ID=w435, data in="3a") -> (connection ID out=w433:refnum<k5>)  [unwired: 2 in, 2 out]
                  n349 = property on="Boolean 31" class="Bool (strict)"("Colors [4]"=cluster{u32, u32}[] [{16777216, 16711680}, {16777216, 16711680}, {16777216, 16711680}, {16777216, 16711680}] ("Colors [4] 2")) -> ()  [unwired: 2 in, 2 out]
                }
              }
            }
            frame "32" {
              n350 = property on="Boolean 32" class="Bool (strict)"() -> ("Colors [4]"=w446:cluster{u32, u32}[])  [unwired: 2 in, 2 out]
              n351 = for {
                N: 1 -> [_]
                tunnel: cluster{u32, u32}[] [{16777216, 32639}, {16777216, 32639}, {16777216, 32639}, {16777216, 32639}] ("Colors [4] 2") -> [w465] mode=indexing
                tunnel: [w463] -> w449
                tunnel: w446 -> [w462] mode=indexing
                n352 = Equal?(x=w462, y=w465) -> (x = y?=w464:cluster{bool, bool})
                n353 = Unbundle(w464) -> (w463:bool)  [unwired: 1 out]
              }
              n354 = case shown="True" w449 {
                tunnel: w448 -> [w455 w461]
                tunnel: [w455 w460] -> w447
                tunnel: w445 -> [w453 w457]
                tunnel: [w452 w456] -> w444
                frame False {
                  n355 = TCP Write(connection ID=w453, data in="b3") -> (connection ID out=w452:refnum<k5>)  [unwired: 2 in, 2 out]
                }
                frame True {
                  n356 = Increment(x=w461) -> (x+1=w460:i32)
                  n357 = TCP Write(connection ID=w457, data in="3b") -> (connection ID out=w456:refnum<k5>)  [unwired: 2 in, 2 out]
                  n358 = property on="Boolean 32" class="Bool (strict)"("Colors [4]"=cluster{u32, u32}[] [{16777216, 16711680}, {16777216, 16711680}, {16777216, 16711680}, {16777216, 16711680}] ("Colors [4] 2")) -> ()  [unwired: 2 in, 2 out]
                }
              }
            }
            frame "33" {
              n359 = property on="Boolean 33" class="Bool (strict)"() -> ("Colors [4]"=w469:cluster{u32, u32}[])  [unwired: 2 in, 2 out]
              n360 = for {
                N: 1 -> [_]
                tunnel: cluster{u32, u32}[] [{16777216, 32639}, {16777216, 32639}, {16777216, 32639}, {16777216, 32639}] ("Colors [4] 2") -> [w488] mode=indexing
                tunnel: [w486] -> w472
                tunnel: w469 -> [w485] mode=indexing
                n361 = Equal?(x=w485, y=w488) -> (x = y?=w487:cluster{bool, bool})
                n362 = Unbundle(w487) -> (w486:bool)  [unwired: 1 out]
              }
              n363 = case shown="True" w472 {
                tunnel: w471 -> [w478 w484]
                tunnel: [w478 w483] -> w470
                tunnel: w468 -> [w476 w480]
                tunnel: [w475 w479] -> w467
                frame False {
                  n364 = TCP Write(connection ID=w476, data in="c3") -> (connection ID out=w475:refnum<k5>)  [unwired: 2 in, 2 out]
                }
                frame True {
                  n365 = Increment(x=w484) -> (x+1=w483:i32)
                  n366 = TCP Write(connection ID=w480, data in="3c") -> (connection ID out=w479:refnum<k5>)  [unwired: 2 in, 2 out]
                  n367 = property on="Boolean 33" class="Bool (strict)"("Colors [4]"=cluster{u32, u32}[] [{16777216, 16711680}, {16777216, 16711680}, {16777216, 16711680}, {16777216, 16711680}] ("Colors [4] 2")) -> ()  [unwired: 2 in, 2 out]
                }
              }
            }
            frame "34" {
              n368 = property on="Boolean 34" class="Bool (strict)"() -> ("Colors [4]"=w492:cluster{u32, u32}[])  [unwired: 2 in, 2 out]
              n369 = for {
                N: 1 -> [_]
                tunnel: cluster{u32, u32}[] [{16777216, 32639}, {16777216, 32639}, {16777216, 32639}, {16777216, 32639}] ("Colors [4] 2") -> [w511] mode=indexing
                tunnel: [w509] -> w495
                tunnel: w492 -> [w508] mode=indexing
                n370 = Equal?(x=w508, y=w511) -> (x = y?=w510:cluster{bool, bool})
                n371 = Unbundle(w510) -> (w509:bool)  [unwired: 1 out]
              }
              n372 = case shown="False" w495 {
                tunnel: w494 -> [w501 w507]
                tunnel: [w501 w506] -> w493
                tunnel: w491 -> [w500 w504]
                tunnel: [w498 w502] -> w490
                frame False {
                  n373 = TCP Write(connection ID=w500, data in="d3") -> (connection ID out=w498:refnum<k5>)  [unwired: 2 in, 2 out]
                }
                frame True {
                  n374 = Increment(x=w507) -> (x+1=w506:i32)
                  n375 = TCP Write(connection ID=w504, data in="3d") -> (connection ID out=w502:refnum<k5>)  [unwired: 2 in, 2 out]
                  n376 = property on="Boolean 34" class="Bool (strict)"("Colors [4]"=cluster{u32, u32}[] [{16777216, 16711680}, {16777216, 16711680}, {16777216, 16711680}, {16777216, 16711680}] ("Colors [4] 2")) -> ()  [unwired: 2 in, 2 out]
                }
              }
            }
            frame "35" {
              n377 = property on="Boolean 35" class="Bool (strict)"() -> ("Colors [4]"=w515:cluster{u32, u32}[])  [unwired: 2 in, 2 out]
              n378 = for {
                N: 1 -> [_]
                tunnel: cluster{u32, u32}[] [{16777216, 32639}, {16777216, 32639}, {16777216, 32639}, {16777216, 32639}] ("Colors [4] 2") -> [w534] mode=indexing
                tunnel: [w532] -> w518
                tunnel: w515 -> [w531] mode=indexing
                n379 = Equal?(x=w531, y=w534) -> (x = y?=w533:cluster{bool, bool})
                n380 = Unbundle(w533) -> (w532:bool)  [unwired: 1 out]
              }
              n381 = case shown="False" w518 {
                tunnel: w517 -> [w524 w530]
                tunnel: [w524 w529] -> w516
                tunnel: w514 -> [w522 w527]
                tunnel: [w521 w525] -> w513
                frame False {
                  n382 = TCP Write(connection ID=w522, data in="e3") -> (connection ID out=w521:refnum<k5>)  [unwired: 2 in, 2 out]
                }
                frame True {
                  n383 = Increment(x=w530) -> (x+1=w529:i32)
                  n384 = TCP Write(connection ID=w527, data in="3e") -> (connection ID out=w525:refnum<k5>)  [unwired: 2 in, 2 out]
                  n385 = property on="Boolean 35" class="Bool (strict)"("Colors [4]"=cluster{u32, u32}[] [{16777216, 16711680}, {16777216, 16711680}, {16777216, 16711680}, {16777216, 16711680}] ("Colors [4] 2")) -> ()  [unwired: 2 in, 2 out]
                }
              }
            }
            frame "36" {
              n386 = property on="Boolean 36" class="Bool (strict)"() -> ("Colors [4]"=w538:cluster{u32, u32}[])  [unwired: 2 in, 2 out]
              n387 = for {
                N: 1 -> [_]
                tunnel: cluster{u32, u32}[] [{16777216, 32639}, {16777216, 32639}, {16777216, 32639}, {16777216, 32639}] ("Colors [4] 2") -> [w557] mode=indexing
                tunnel: [w555] -> w541
                tunnel: w538 -> [w554] mode=indexing
                n388 = Equal?(x=w554, y=w557) -> (x = y?=w556:cluster{bool, bool})
                n389 = Unbundle(w556) -> (w555:bool)  [unwired: 1 out]
              }
              n390 = case shown="True" w541 {
                tunnel: w540 -> [w547 w553]
                tunnel: [w547 w552] -> w539
                tunnel: w537 -> [w545 w549]
                tunnel: [w544 w548] -> w536
                frame False {
                  n391 = TCP Write(connection ID=w545, data in="f3") -> (connection ID out=w544:refnum<k5>)  [unwired: 2 in, 2 out]
                }
                frame True {
                  n392 = Increment(x=w553) -> (x+1=w552:i32)
                  n393 = TCP Write(connection ID=w549, data in="3f") -> (connection ID out=w548:refnum<k5>)  [unwired: 2 in, 2 out]
                  n394 = property on="Boolean 36" class="Bool (strict)"("Colors [4]"=cluster{u32, u32}[] [{16777216, 16711680}, {16777216, 16711680}, {16777216, 16711680}, {16777216, 16711680}] ("Colors [4] 2")) -> ()  [unwired: 2 in, 2 out]
                }
              }
            }
            frame "37" {
              n395 = property on="Boolean 37" class="Bool (strict)"() -> ("Colors [4]"=w561:cluster{u32, u32}[])  [unwired: 2 in, 2 out]
              n396 = for {
                N: 1 -> [_]
                tunnel: cluster{u32, u32}[] [{16777216, 32639}, {16777216, 32639}, {16777216, 32639}, {16777216, 32639}] ("Colors [4] 2") -> [w580] mode=indexing
                tunnel: [w578] -> w564
                tunnel: w561 -> [w577] mode=indexing
                n397 = Equal?(x=w577, y=w580) -> (x = y?=w579:cluster{bool, bool})
                n398 = Unbundle(w579) -> (w578:bool)  [unwired: 1 out]
              }
              n399 = case shown="True" w564 {
                tunnel: w563 -> [w570 w576]
                tunnel: [w570 w575] -> w562
                tunnel: w560 -> [w568 w572]
                tunnel: [w569 w571] -> w559
                frame False {
                  n400 = TCP Write(connection ID=w568, data in="g3") -> (connection ID out=w569:refnum<k5>)  [unwired: 2 in, 2 out]
                }
                frame True {
                  n401 = TCP Write(connection ID=w572, data in="3g") -> (connection ID out=w571:refnum<k5>)  [unwired: 2 in, 2 out]
                  n402 = property on="Boolean 37" class="Bool (strict)"("Colors [4]"=cluster{u32, u32}[] [{16777216, 16711680}, {16777216, 16711680}, {16777216, 16711680}, {16777216, 16711680}] ("Colors [4] 2")) -> ()  [unwired: 2 in, 2 out]
                  n403 = Increment(x=w576) -> (x+1=w575:i32)
                }
              }
            }
            frame "38" {
              n404 = property on="Boolean 38" class="Bool (strict)"() -> ("Colors [4]"=w584:cluster{u32, u32}[])  [unwired: 2 in, 2 out]
              n405 = for {
                N: 1 -> [_]
                tunnel: cluster{u32, u32}[] [{16777216, 32639}, {16777216, 32639}, {16777216, 32639}, {16777216, 32639}] ("Colors [4] 2") -> [w603] mode=indexing
                tunnel: [w601] -> w587
                tunnel: w584 -> [w600] mode=indexing
                n406 = Equal?(x=w600, y=w603) -> (x = y?=w602:cluster{bool, bool})
                n407 = Unbundle(w602) -> (w601:bool)  [unwired: 1 out]
              }
              n408 = case shown="True" w587 {
                tunnel: w586 -> [w593 w599]
                tunnel: [w593 w598] -> w585
                tunnel: w583 -> [w592 w595]
                tunnel: [w590 w594] -> w582
                frame False {
                  n409 = TCP Write(connection ID=w592, data in="h3") -> (connection ID out=w590:refnum<k5>)  [unwired: 2 in, 2 out]
                }
                frame True {
                  n410 = TCP Write(connection ID=w595, data in="3h") -> (connection ID out=w594:refnum<k5>)  [unwired: 2 in, 2 out]
                  n411 = property on="Boolean 38" class="Bool (strict)"("Colors [4]"=cluster{u32, u32}[] [{16777216, 16711680}, {16777216, 16711680}, {16777216, 16711680}, {16777216, 16711680}] ("Colors [4] 2")) -> ()  [unwired: 2 in, 2 out]
                  n412 = Increment(x=w599) -> (x+1=w598:i32)
                }
              }
            }
            frame "39" {
              n413 = property on="Boolean 39" class="Bool (strict)"() -> ("Colors [4]"=w607:cluster{u32, u32}[])  [unwired: 2 in, 2 out]
              n414 = for {
                N: 1 -> [_]
                tunnel: cluster{u32, u32}[] [{16777216, 32639}, {16777216, 32639}, {16777216, 32639}, {16777216, 32639}] ("Colors [4] 2") -> [w626] mode=indexing
                tunnel: [w624] -> w610
                tunnel: w607 -> [w623] mode=indexing
                n415 = Equal?(x=w623, y=w626) -> (x = y?=w625:cluster{bool, bool})
                n416 = Unbundle(w625) -> (w624:bool)  [unwired: 1 out]
              }
              n417 = case shown="True" w610 {
                tunnel: w609 -> [w616 w622]
                tunnel: [w616 w621] -> w608
                tunnel: w606 -> [w614 w618]
                tunnel: [w613 w617] -> w605
                frame False {
                  n418 = TCP Write(connection ID=w614, data in="i3") -> (connection ID out=w613:refnum<k5>)  [unwired: 2 in, 2 out]
                }
                frame True {
                  n419 = TCP Write(connection ID=w618, data in="3i") -> (connection ID out=w617:refnum<k5>)  [unwired: 2 in, 2 out]
                  n420 = property on="Boolean 39" class="Bool (strict)"("Colors [4]"=cluster{u32, u32}[] [{16777216, 16711680}, {16777216, 16711680}, {16777216, 16711680}, {16777216, 16711680}] ("Colors [4] 2")) -> ()  [unwired: 2 in, 2 out]
                  n421 = Increment(x=w622) -> (x+1=w621:i32)
                }
              }
            }
            frame "40" {
              n422 = property on="Boolean 40" class="Bool (strict)"() -> ("Colors [4]"=w630:cluster{u32, u32}[])  [unwired: 2 in, 2 out]
              n423 = for {
                N: 1 -> [_]
                tunnel: cluster{u32, u32}[] [{16777216, 32639}, {16777216, 32639}, {16777216, 32639}, {16777216, 32639}] ("Colors [4] 2") -> [w649] mode=indexing
                tunnel: [w647] -> w633
                tunnel: w630 -> [w646] mode=indexing
                n424 = Equal?(x=w646, y=w649) -> (x = y?=w648:cluster{bool, bool})
                n425 = Unbundle(w648) -> (w647:bool)  [unwired: 1 out]
              }
              n426 = case shown="True" w633 {
                tunnel: w632 -> [w639 w645]
                tunnel: [w639 w644] -> w631
                tunnel: w629 -> [w637 w641]
                tunnel: [w636 w640] -> w628
                frame False {
                  n427 = TCP Write(connection ID=w637, data in="j4") -> (connection ID out=w636:refnum<k5>)  [unwired: 2 in, 2 out]
                }
                frame True {
                  n428 = TCP Write(connection ID=w641, data in="4j") -> (connection ID out=w640:refnum<k5>)  [unwired: 2 in, 2 out]
                  n429 = property on="Boolean 40" class="Bool (strict)"("Colors [4]"=cluster{u32, u32}[] [{16777216, 16711680}, {16777216, 16711680}, {16777216, 16711680}, {16777216, 16711680}] ("Colors [4] 2")) -> ()  [unwired: 2 in, 2 out]
                  n430 = Increment(x=w645) -> (x+1=w644:i32)
                }
              }
            }
            frame "41" {
              n431 = property on="Boolean 41" class="Bool (strict)"() -> ("Colors [4]"=w653:cluster{u32, u32}[])  [unwired: 2 in, 2 out]
              n432 = for {
                N: 1 -> [_]
                tunnel: cluster{u32, u32}[] [{16777216, 32639}, {16777216, 32639}, {16777216, 32639}, {16777216, 32639}] ("Colors [4] 2") -> [w672] mode=indexing
                tunnel: [w670] -> w656
                tunnel: w653 -> [w669] mode=indexing
                n433 = Equal?(x=w669, y=w672) -> (x = y?=w671:cluster{bool, bool})
                n434 = Unbundle(w671) -> (w670:bool)  [unwired: 1 out]
              }
              n435 = case shown="False" w656 {
                tunnel: w655 -> [w662 w668]
                tunnel: [w662 w667] -> w654
                tunnel: w652 -> [w660 w664]
                tunnel: [w659 w663] -> w651
                frame False {
                  n436 = TCP Write(connection ID=w660, data in="a4") -> (connection ID out=w659:refnum<k5>)  [unwired: 2 in, 2 out]
                }
                frame True {
                  n437 = TCP Write(connection ID=w664, data in="4a") -> (connection ID out=w663:refnum<k5>)  [unwired: 2 in, 2 out]
                  n438 = property on="Boolean 41" class="Bool (strict)"("Colors [4]"=cluster{u32, u32}[] [{16777216, 16711680}, {16777216, 16711680}, {16777216, 16711680}, {16777216, 16711680}] ("Colors [4] 2")) -> ()  [unwired: 2 in, 2 out]
                  n439 = Increment(x=w668) -> (x+1=w667:i32)
                }
              }
            }
            frame "42" {
              n440 = property on="Boolean 42" class="Bool (strict)"() -> ("Colors [4]"=w676:cluster{u32, u32}[])  [unwired: 2 in, 2 out]
              n441 = for {
                N: 1 -> [_]
                tunnel: cluster{u32, u32}[] [{16777216, 32639}, {16777216, 32639}, {16777216, 32639}, {16777216, 32639}] ("Colors [4] 2") -> [w695] mode=indexing
                tunnel: [w693] -> w679
                tunnel: w676 -> [w692] mode=indexing
                n442 = Equal?(x=w692, y=w695) -> (x = y?=w694:cluster{bool, bool})
                n443 = Unbundle(w694) -> (w693:bool)  [unwired: 1 out]
              }
              n444 = case shown="True" w679 {
                tunnel: w678 -> [w685 w691]
                tunnel: [w685 w690] -> w677
                tunnel: w675 -> [w683 w687]
                tunnel: [w682 w686] -> w674
                frame False {
                  n445 = TCP Write(connection ID=w683, data in="b4") -> (connection ID out=w682:refnum<k5>)  [unwired: 2 in, 2 out]
                }
                frame True {
                  n446 = TCP Write(connection ID=w687, data in="4b") -> (connection ID out=w686:refnum<k5>)  [unwired: 2 in, 2 out]
                  n447 = property on="Boolean 42" class="Bool (strict)"("Colors [4]"=cluster{u32, u32}[] [{16777216, 16711680}, {16777216, 16711680}, {16777216, 16711680}, {16777216, 16711680}] ("Colors [4] 2")) -> ()  [unwired: 2 in, 2 out]
                  n448 = Increment(x=w691) -> (x+1=w690:i32)
                }
              }
            }
            frame "43" {
              n449 = property on="Boolean 43" class="Bool (strict)"() -> ("Colors [4]"=w699:cluster{u32, u32}[])  [unwired: 2 in, 2 out]
              n450 = for {
                N: 1 -> [_]
                tunnel: cluster{u32, u32}[] [{16777216, 32639}, {16777216, 32639}, {16777216, 32639}, {16777216, 32639}] ("Colors [4] 2") -> [w718] mode=indexing
                tunnel: [w716] -> w702
                tunnel: w699 -> [w715] mode=indexing
                n451 = Equal?(x=w715, y=w718) -> (x = y?=w717:cluster{bool, bool})
                n452 = Unbundle(w717) -> (w716:bool)  [unwired: 1 out]
              }
              n453 = case shown="False" w702 {
                tunnel: w701 -> [w708 w714]
                tunnel: [w708 w713] -> w700
                tunnel: w698 -> [w706 w710]
                tunnel: [w705 w709] -> w697
                frame False {
                  n454 = TCP Write(connection ID=w706, data in="c4") -> (connection ID out=w705:refnum<k5>)  [unwired: 2 in, 2 out]
                }
                frame True {
                  n455 = TCP Write(connection ID=w710, data in="4c") -> (connection ID out=w709:refnum<k5>)  [unwired: 2 in, 2 out]
                  n456 = property on="Boolean 43" class="Bool (strict)"("Colors [4]"=cluster{u32, u32}[] [{16777216, 16711680}, {16777216, 16711680}, {16777216, 16711680}, {16777216, 16711680}] ("Colors [4] 2")) -> ()  [unwired: 2 in, 2 out]
                  n457 = Increment(x=w714) -> (x+1=w713:i32)
                }
              }
            }
            frame "44" {
              n458 = property on="Boolean 44" class="Bool (strict)"() -> ("Colors [4]"=w722:cluster{u32, u32}[])  [unwired: 2 in, 2 out]
              n459 = for {
                N: 1 -> [_]
                tunnel: cluster{u32, u32}[] [{16777216, 32639}, {16777216, 32639}, {16777216, 32639}, {16777216, 32639}] ("Colors [4] 2") -> [w741] mode=indexing
                tunnel: [w739] -> w725
                tunnel: w722 -> [w738] mode=indexing
                n460 = Equal?(x=w738, y=w741) -> (x = y?=w740:cluster{bool, bool})
                n461 = Unbundle(w740) -> (w739:bool)  [unwired: 1 out]
              }
              n462 = case shown="True" w725 {
                tunnel: w724 -> [w731 w737]
                tunnel: [w731 w736] -> w723
                tunnel: w721 -> [w729 w733]
                tunnel: [w728 w732] -> w720
                frame False {
                  n463 = TCP Write(connection ID=w729, data in="d4") -> (connection ID out=w728:refnum<k5>)  [unwired: 2 in, 2 out]
                }
                frame True {
                  n464 = TCP Write(connection ID=w733, data in="4d") -> (connection ID out=w732:refnum<k5>)  [unwired: 2 in, 2 out]
                  n465 = property on="Boolean 44" class="Bool (strict)"("Colors [4]"=cluster{u32, u32}[] [{16777216, 16711680}, {16777216, 16711680}, {16777216, 16711680}, {16777216, 16711680}] ("Colors [4] 2")) -> ()  [unwired: 2 in, 2 out]
                  n466 = Increment(x=w737) -> (x+1=w736:i32)
                }
              }
            }
            frame "45" {
              n467 = property on="Boolean 45" class="Bool (strict)"() -> ("Colors [4]"=w745:cluster{u32, u32}[])  [unwired: 2 in, 2 out]
              n468 = for {
                N: 1 -> [_]
                tunnel: cluster{u32, u32}[] [{16777216, 32639}, {16777216, 32639}, {16777216, 32639}, {16777216, 32639}] ("Colors [4] 2") -> [w764] mode=indexing
                tunnel: [w762] -> w748
                tunnel: w745 -> [w761] mode=indexing
                n469 = Equal?(x=w761, y=w764) -> (x = y?=w763:cluster{bool, bool})
                n470 = Unbundle(w763) -> (w762:bool)  [unwired: 1 out]
              }
              n471 = case shown="True" w748 {
                tunnel: w747 -> [w754 w760]
                tunnel: [w754 w759] -> w746
                tunnel: w744 -> [w753 w756]
                tunnel: [w751 w755] -> w743
                frame False {
                  n472 = TCP Write(connection ID=w753, data in="e4") -> (connection ID out=w751:refnum<k5>)  [unwired: 2 in, 2 out]
                }
                frame True {
                  n473 = TCP Write(connection ID=w756, data in="4e") -> (connection ID out=w755:refnum<k5>)  [unwired: 2 in, 2 out]
                  n474 = property on="Boolean 45" class="Bool (strict)"("Colors [4]"=cluster{u32, u32}[] [{16777216, 16711680}, {16777216, 16711680}, {16777216, 16711680}, {16777216, 16711680}] ("Colors [4] 2")) -> ()  [unwired: 2 in, 2 out]
                  n475 = Increment(x=w760) -> (x+1=w759:i32)
                }
              }
            }
            frame "46" {
              n476 = property on="Boolean 46" class="Bool (strict)"() -> ("Colors [4]"=w768:cluster{u32, u32}[])  [unwired: 2 in, 2 out]
              n477 = for {
                N: 1 -> [_]
                tunnel: cluster{u32, u32}[] [{16777216, 32639}, {16777216, 32639}, {16777216, 32639}, {16777216, 32639}] ("Colors [4] 2") -> [w787] mode=indexing
                tunnel: [w785] -> w771
                tunnel: w768 -> [w784] mode=indexing
                n478 = Equal?(x=w784, y=w787) -> (x = y?=w786:cluster{bool, bool})
                n479 = Unbundle(w786) -> (w785:bool)  [unwired: 1 out]
              }
              n480 = case shown="True" w771 {
                tunnel: w770 -> [w777 w783]
                tunnel: [w777 w782] -> w769
                tunnel: w767 -> [w776 w779]
                tunnel: [w774 w778] -> w766
                frame False {
                  n481 = TCP Write(connection ID=w776, data in="f4") -> (connection ID out=w774:refnum<k5>)  [unwired: 2 in, 2 out]
                }
                frame True {
                  n482 = TCP Write(connection ID=w779, data in="4f") -> (connection ID out=w778:refnum<k5>)  [unwired: 2 in, 2 out]
                  n483 = property on="Boolean 46" class="Bool (strict)"("Colors [4]"=cluster{u32, u32}[] [{16777216, 16711680}, {16777216, 16711680}, {16777216, 16711680}, {16777216, 16711680}] ("Colors [4] 2")) -> ()  [unwired: 2 in, 2 out]
                  n484 = Increment(x=w783) -> (x+1=w782:i32)
                }
              }
            }
            frame "47" {
              n485 = property on="Boolean 47" class="Bool (strict)"() -> ("Colors [4]"=w791:cluster{u32, u32}[])  [unwired: 2 in, 2 out]
              n486 = for {
                N: 1 -> [_]
                tunnel: cluster{u32, u32}[] [{16777216, 32639}, {16777216, 32639}, {16777216, 32639}, {16777216, 32639}] ("Colors [4] 2") -> [w810] mode=indexing
                tunnel: [w808] -> w794
                tunnel: w791 -> [w807] mode=indexing
                n487 = Equal?(x=w807, y=w810) -> (x = y?=w809:cluster{bool, bool})
                n488 = Unbundle(w809) -> (w808:bool)  [unwired: 1 out]
              }
              n489 = case shown="True" w794 {
                tunnel: w793 -> [w800 w806]
                tunnel: [w800 w805] -> w792
                tunnel: w790 -> [w798 w802]
                tunnel: [w797 w801] -> w789
                frame False {
                  n490 = TCP Write(connection ID=w798, data in="g4") -> (connection ID out=w797:refnum<k5>)  [unwired: 2 in, 2 out]
                }
                frame True {
                  n491 = TCP Write(connection ID=w802, data in="4g") -> (connection ID out=w801:refnum<k5>)  [unwired: 2 in, 2 out]
                  n492 = property on="Boolean 47" class="Bool (strict)"("Colors [4]"=cluster{u32, u32}[] [{16777216, 16711680}, {16777216, 16711680}, {16777216, 16711680}, {16777216, 16711680}] ("Colors [4] 2")) -> ()  [unwired: 2 in, 2 out]
                  n493 = Increment(x=w806) -> (x+1=w805:i32)
                }
              }
            }
            frame "48" {
              n494 = property on="Boolean 48" class="Bool (strict)"() -> ("Colors [4]"=w814:cluster{u32, u32}[])  [unwired: 2 in, 2 out]
              n495 = for {
                N: 1 -> [_]
                tunnel: cluster{u32, u32}[] [{16777216, 32639}, {16777216, 32639}, {16777216, 32639}, {16777216, 32639}] ("Colors [4] 2") -> [w833] mode=indexing
                tunnel: [w831] -> w817
                tunnel: w814 -> [w830] mode=indexing
                n496 = Equal?(x=w830, y=w833) -> (x = y?=w832:cluster{bool, bool})
                n497 = Unbundle(w832) -> (w831:bool)  [unwired: 1 out]
              }
              n498 = case shown="False" w817 {
                tunnel: w816 -> [w823 w829]
                tunnel: [w823 w828] -> w815
                tunnel: w813 -> [w821 w825]
                tunnel: [w820 w824] -> w812
                frame False {
                  n499 = TCP Write(connection ID=w821, data in="h4") -> (connection ID out=w820:refnum<k5>)  [unwired: 2 in, 2 out]
                }
                frame True {
                  (unwired) u16 82 ("port")
                  n500 = TCP Write(connection ID=w825, data in="4h") -> (connection ID out=w824:refnum<k5>)  [unwired: 2 in, 2 out]
                  n501 = property on="Boolean 48" class="Bool (strict)"("Colors [4]"=cluster{u32, u32}[] [{16777216, 16711680}, {16777216, 16711680}, {16777216, 16711680}, {16777216, 16711680}] ("Colors [4] 2")) -> ()  [unwired: 2 in, 2 out]
                  n502 = Increment(x=w829) -> (x+1=w828:i32)
                }
              }
            }
            frame "49" {
              n503 = property on="Boolean 49" class="Bool (strict)"() -> ("Colors [4]"=w837:cluster{u32, u32}[])  [unwired: 2 in, 2 out]
              n504 = for {
                N: 1 -> [_]
                tunnel: cluster{u32, u32}[] [{16777216, 32639}, {16777216, 32639}, {16777216, 32639}, {16777216, 32639}] ("Colors [4] 2") -> [w856] mode=indexing
                tunnel: [w854] -> w840
                tunnel: w837 -> [w853] mode=indexing
                n505 = Equal?(x=w853, y=w856) -> (x = y?=w855:cluster{bool, bool})
                n506 = Unbundle(w855) -> (w854:bool)  [unwired: 1 out]
              }
              n507 = case shown="False" w840 {
                tunnel: w839 -> [w846 w852]
                tunnel: [w846 w851] -> w838
                tunnel: w836 -> [w845 w848]
                tunnel: [w844 w847] -> w835
                frame False {
                  n508 = TCP Write(connection ID=w845, data in="i4") -> (connection ID out=w844:refnum<k5>)  [unwired: 2 in, 2 out]
                }
                frame True {
                  n509 = TCP Write(connection ID=w848, data in="4i") -> (connection ID out=w847:refnum<k5>)  [unwired: 2 in, 2 out]
                  n510 = Increment(x=w852) -> (x+1=w851:i32)
                  n511 = property on="Boolean 49" class="Bool (strict)"("Colors [4]"=cluster{u32, u32}[] [{16777216, 16711680}, {16777216, 16711680}, {16777216, 16711680}, {16777216, 16711680}] ("Colors [4] 2")) -> ()  [unwired: 2 in, 2 out]
                }
              }
            }
            frame "50" {
              n512 = property on="Boolean 50" class="Bool (strict)"() -> ("Colors [4]"=w860:cluster{u32, u32}[])  [unwired: 2 in, 2 out]
              n513 = for {
                N: 1 -> [_]
                tunnel: cluster{u32, u32}[] [{16777216, 32639}, {16777216, 32639}, {16777216, 32639}, {16777216, 32639}] ("Colors [4] 2") -> [w879] mode=indexing
                tunnel: [w877] -> w863
                tunnel: w860 -> [w876] mode=indexing
                n514 = Equal?(x=w876, y=w879) -> (x = y?=w878:cluster{bool, bool})
                n515 = Unbundle(w878) -> (w877:bool)  [unwired: 1 out]
              }
              n516 = case shown="True" w863 {
                tunnel: w862 -> [w869 w875]
                tunnel: [w869 w874] -> w861
                tunnel: w859 -> [w867 w871]
                tunnel: [w866 w870] -> w858
                frame False {
                  n517 = TCP Write(connection ID=w867, data in="j5") -> (connection ID out=w866:refnum<k5>)  [unwired: 2 in, 2 out]
                }
                frame True {
                  n518 = TCP Write(connection ID=w871, data in="5j") -> (connection ID out=w870:refnum<k5>)  [unwired: 2 in, 2 out]
                  n519 = Increment(x=w875) -> (x+1=w874:i32)
                  n520 = property on="Boolean 50" class="Bool (strict)"("Colors [4]"=cluster{u32, u32}[] [{16777216, 16711680}, {16777216, 16711680}, {16777216, 16711680}, {16777216, 16711680}] ("Colors [4] 2")) -> ()  [unwired: 2 in, 2 out]
                }
              }
            }
            frame "vv" {
              n521 = TCP Close Connection(connection ID=w881) -> ()  [unwired: 2 in, 2 out]
              n522 = TCP Close Connection(connection ID=w882) -> ()  [unwired: 2 in, 2 out]
              n523 = property on="String" class="Str"("Value"="You win") -> ()  [unwired: 2 in, 2 out]
            }
          }
          n524 = Greater?(x=w99, y=5) -> (0:w95:bool)
          n525 = Or(x=w95, y=w96) -> (x .or. y?=w89:bool)
          n526 = case shown="True" w95 {
            tunnel: w93 -> [_ w888]
            tunnel: w97 -> [_ w886]
            frame False {
            }
            frame True {
              n527 = TCP Close Connection(connection ID=w888) -> ()  [unwired: 2 in, 2 out]
              n528 = property on="String" class="Str"("Value"="You lose") -> ()  [unwired: 2 in, 2 out]
              n529 = TCP Write(connection ID=w886, data in="vv") -> (connection ID out=w885:refnum<k5>)  [unwired: 2 in, 2 out]
              n530 = TCP Close Connection(connection ID=w885) -> ()  [unwired: 2 in, 2 out]
            }
          }
        }
      }
    }
  }
